vi "Camber controller April 18 2016.vi"() -> ()   [LabVIEW 2014]
uses:
  <vilib>/Utility/error.llb/DialogType.ctl
  <vilib>/Instr/_visa.llb/VISA Configure Serial Port (Instr).vi
  <vilib>/Utility/file.llb/Write To Spreadsheet File (string).vi
  <vilib>/Utility/file.llb/Write To Spreadsheet File (DBL).vi
  <vilib>/Utility/file.llb/Read From Spreadsheet File (string).vi
  <vilib>/DAQmx/read.llb/DAQmx Read (Analog 1D DBL NChan 1Samp).vi
  <vilib>/DAQmx/write.llb/DAQmx Write (Analog 1D DBL NChan 1Samp).vi
  <vilib>/DAQmx/write.llb/DAQmx Write (Digital Bool 1Line 1Point).vi
  Environmental Chamber LabVIEW and Instruments/Drivers and Software/keithley_6430/Keithley 6430/Public/Data/Read (Single Point).vi
  Environmental Chamber LabVIEW and Instruments/Drivers and Software/LabVIEW 8.2 Drivers/keithley_24xx/Keithley 24XX/Public/Data/Read (Single Point).vi
  Environmental Chamber LabVIEW and Instruments/Drivers and Software/keithley_24xx/Keithley 24XX/Keithley 24XX.lvlib
  Environmental Chamber LabVIEW and Instruments/Drivers and Software/keithley_6430/Keithley 6430/Keithley 6430.lvlib
  LabVIEW QCM code version 4 Working/(SubVI)2 2QCM.vi
  LabVIEW QCM code version 4 Working/(SubVI)1 3QCM.vi
  LabVIEW QCM code version 4 Working/(SubVI)2 3QCM.vi
  LabVIEW QCM code version 4 Working/(SubVI)1 4QCM.vi
  LabVIEW QCM code version 4 Working/(SubVI)2 4QCM.vi
  LabVIEW QCM code version 4 Working/(SubVI)1 5QCM.vi
  LabVIEW QCM code version 4 Working/(SubVI)2 5QCM.vi
  LabVIEW QCM code version 4 Working/(SubVI)1 6QCM.vi
  LabVIEW QCM code version 4 Working/(SubVI)2 6QCM.vi
panel:
  out "Sequence\npreview":cluster{dbl[], dbl[]}[](graph)
  in  "Gate time":u16(ring)=1 items=["0.1 seconds", "1.0 seconds", "10.0 seconds"]
  out "Hz":dbl format="%.2f"
  out "Waveform Chart 2":T1(graph)
  in  "User-defined\nsequence":string[][](table) caption="Create sequence"
  out "Sequence end time":string
  in  "Run Sequence":bool
  in  "Import sequence file":bool
  in  "Save sequence":bool
  in  "Clear sequence":bool
  out "arduino qcm 6":cluster{"Mean":dbl}(graph)
  out "arduino qcm 5":cluster{"Mean":dbl}(graph)
  out "arduino qcm 4":cluster{"Mean":dbl}(graph)
  out "arduino qcm 1":cluster{"Mean":dbl}(graph)
  out "arduino qcm 3":cluster{"Mean":dbl}(graph)
  out "arduino qcm 2":cluster{"Mean":dbl}(graph)
  in  "electrical/optical tab":enum32{"Electrical", "Optical"}(tab)
  out "Keithley 6430 (Ohm)":cluster{"Measurement":dbl}(graph)
  out "Keithley 2420 (Ohm)":cluster{"Resistance":sgl}(graph)
  in  "Seconds between  spectra":dbl caption="Time Target (s)"
  in  "Save spectra file path":path=path "C:/Users/User/Desktop/Chamber Data/perovskites/2015-08-04 spectra"
  in  "spectra settings":i32[](array[numeric]) caption="Integration time (ms)\n\nOptical smoothing level\n\nNumber of scans to average\n\nDigitizer clock rate setting" min=0 max=4 step=1
  in  "Aquire spectra":bool
  out "Critical Error":bool
  out "output param":i32
  out "Spectrum":cluster{"Wavelengths":dbl[], "buffer out":sgl[]}(graph)
  in  "Analyte part. press. (%)":dbl=100.0 min=0.0 max=100.0 step=5.0
  in  "Pressure Mode":T2(radio)
  in  "Turbo pump auto on":bool=TRUE
  in  "Gas sccm":sgl min=0 max=200 step=5
  out "Actual vapor flow":dbl format="%#_3g"
  out "actual gas flow":dbl format="%#_3g"
  in  "Vapor sccm":sgl min=0 max=200 step=5
  in  "Valve":enum32{"% Open", "Torr "}(radio)
  out "Valve position (%)":dbl format="%#_2f"
  in  "Desired pressure":dbl min=0.0 max=760.0 step=5.0
  in  "valve % open":dbl=100.0 min=0.0 max=100.0 step=5.0 format="%#_2f"
  out "actual pressure":dbl format="%#_3g"
  out "Currently saving data":bool
  in  "Data saving":T3(radio)
  out "J-Kem Temp (C)":cluster{"Numeric Control":dbl}(graph)
  out "Chamber Pressure (Torr)":cluster{"f":dbl}(graph)
  in  "Start saving after":dbl caption="min"
  in  "Auto stop after":bool
  in  "hrs":dbl=1000.0 min=0.0
  out "Start Time":string
  out "Elapsed (min)":dbl caption="Elapsed Time (s)" format="%#_4g"
  in  "Delay between data points (s)":dbl caption="sec" min=0.0 max=30.0 format="%#_13g"
  in  "stop":bool
  in  "Experiment Notes":string
  in  "Clear all charts":bool
  out "Data file save path":path
  out "Array for Mean 7":dbl[](array[numeric]) format="%#_8g"
  out "Array for Median 7":dbl[](array[numeric]) format="%#_8g"
  out "Mean 7":dbl format="%#_8g"
  out "Median 7":dbl format="%#_8g"
  out "Array for Mean 6":dbl[](array[numeric]) format="%#_8g"
  out "Array for Median 6":dbl[](array[numeric]) format="%#_8g"
  out "Mean 6":dbl format="%#_8g"
  out "Median 6":dbl format="%#_8g"
  out "Array for Mean 5":dbl[](array[numeric]) format="%#_8g"
  out "Array for Median 5":dbl[](array[numeric]) format="%#_8g"
  out "Mean 5":dbl format="%#_8g"
  out "Median 5":dbl format="%#_8g"
  out "Array for Mean 4":dbl[](array[numeric]) format="%#_8g"
  out "Array for Median 4":dbl[](array[numeric]) format="%#_8g"
  out "Mean 4":dbl format="%#_8g"
  out "Median 4":dbl format="%#_8g"
  out "Array for Mean 3":dbl[](array[numeric]) format="%#_8g"
  out "Array for Median 3":dbl[](array[numeric]) format="%#_8g"
  out "Mean 3":dbl format="%#_8g"
  out "Median 3":dbl format="%#_8g"
  out "Array for Mean 2":dbl[](array[numeric]) format="%#_8g"
  out "Array for Median 2":dbl[](array[numeric]) format="%#_8g"
  out "Mean 2":dbl format="%#_8g"
  out "Median 2":dbl format="%#_8g"
  out "appended array":dbl[](array[numeric]) caption="atm\nTorr"
  in  "rapidox O2 Sensor":bool
  in  "setnag O2 Pump":bool
  in  "Baud Rate 2":i32(ring)=2 items=["2400", "4800", "9600", "19200", "38400", "57600", "115200"]
  in  "Com Port":i32(ring) items=["Com 1", "Com 2", "Com 3", "Com 4", "Com 5", "Com 6", "COM 7", "COM 8", "COM 9", "COM 10", "COM 11", "COM 12", "com 13", "COM 14"]
  in  "Com Port 2":i32(ring) items=["Com 1", "Com 2", "Com 3", "Com 4", "Com 5", "Com 6", "COM 7", "COM 8", "COM 9", "COM 10", "COM 11", "COM 12", "com 13", "COM 14"]
  out "Waveform Chart":cluster{dbl}(graph)
  out "O2 Concentration (PPM)":dbl
  out "Waveform Chart 6":cluster{dbl}(graph)
  # "Currently Unused"
  # "Gas/Vapor Sequence"
  # "Pressure Control"
  # "Actual"
  # "Set"
  # "SRS QCM"
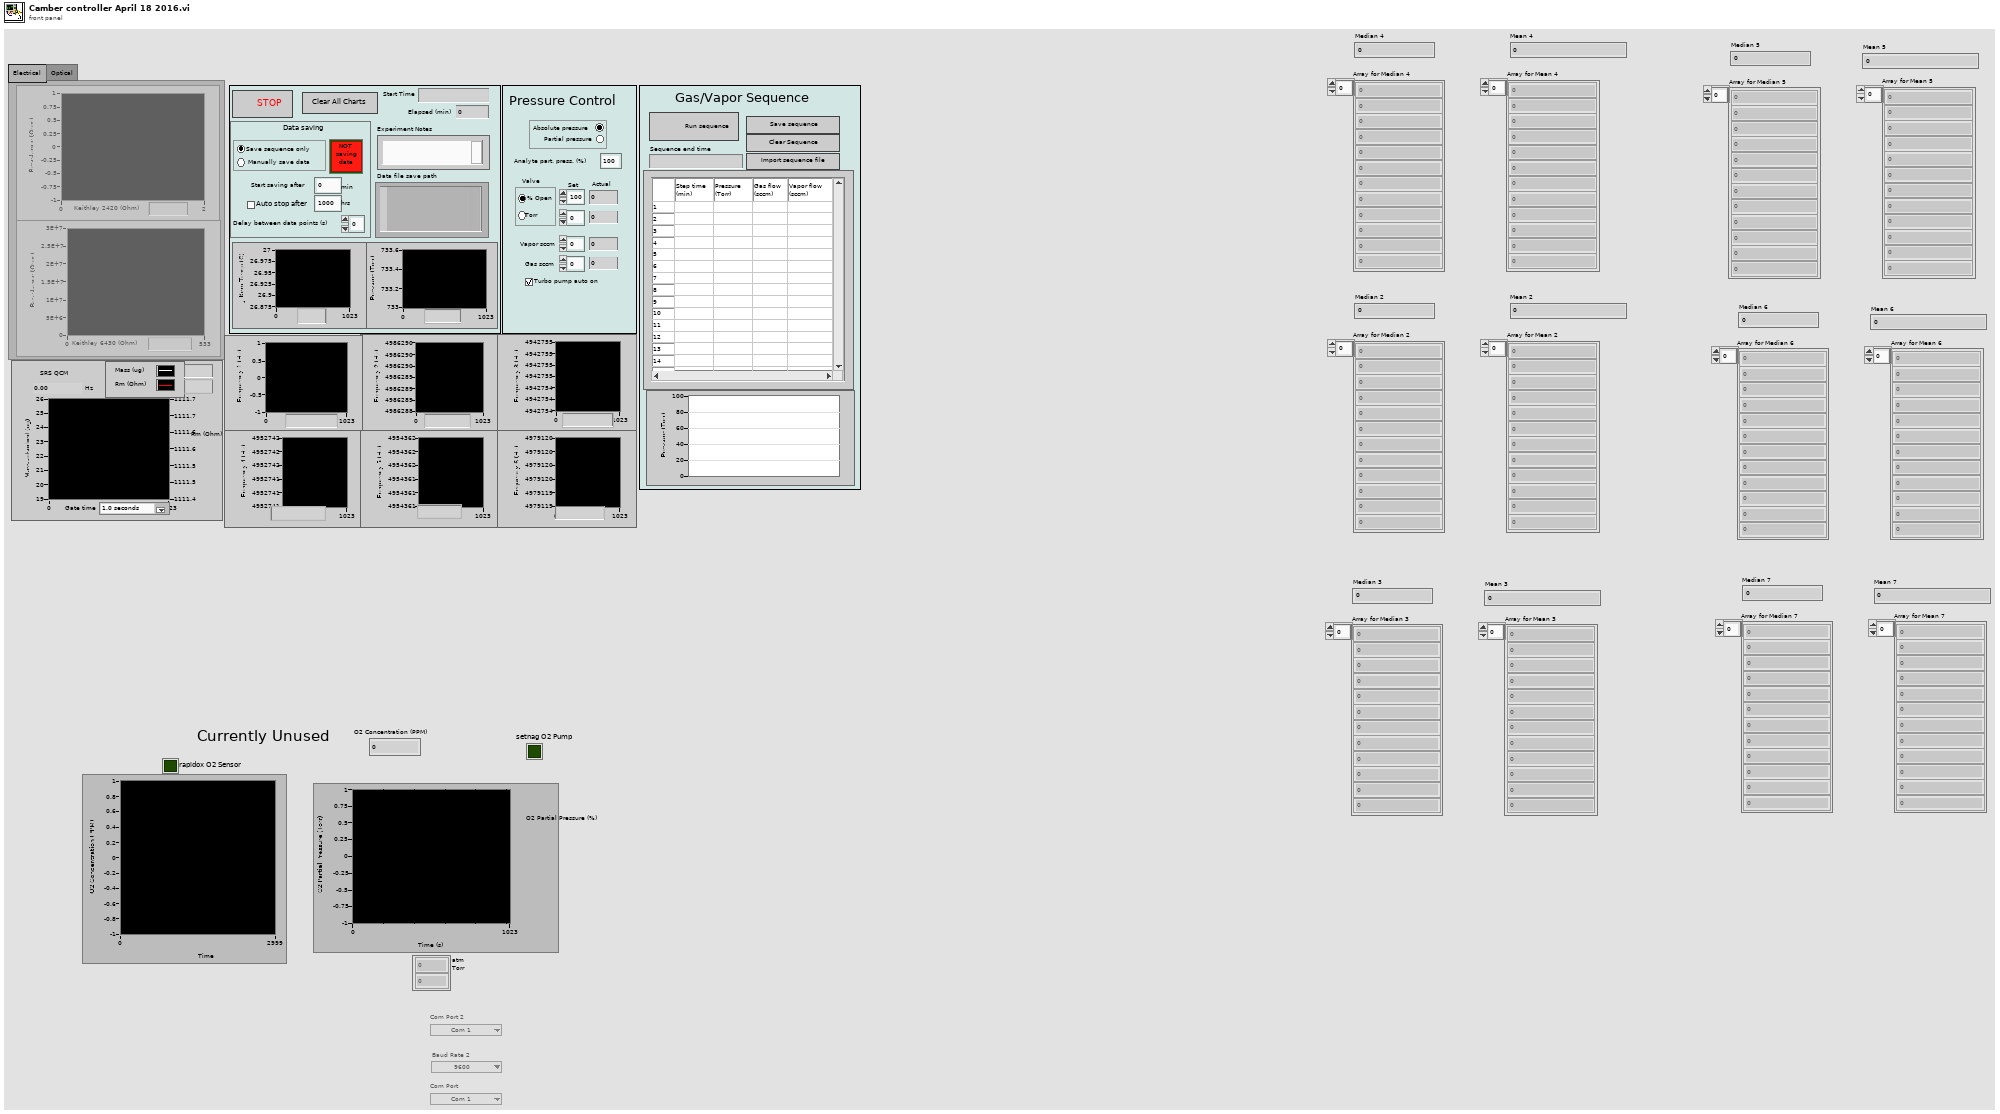
[diagram p1: front panel]
types:
  T1 = cluster{"Numeric Control":dbl, "Resistance out":dbl}
  T2 = enum32{"Absolute pressure ", " Partial pressure"}
  T3 = enum32{"Save sequence only", " Manually save data"}
  T4 = enum16{"open", "open or create", "create or replace", "create", "open (read only)"}
  T5 = enum8{"Enabled", "Disabled", "Disabled and Grayed Out"}
  T6 = enum16{"no parity", "odd parity", "even parity", "mark parity", "space parity"}
  T7 = cluster{"task out":refnum<k21>, "error out":errorcluster, "task out":refnum<k21>, "error out":errorcluster, "task out":refnum<k21>, "error out":errorcluster, "VISA resource name":refnum<visa-resource-name>, "error out":errorcluster}
  T8 = cluster{"task out":refnum<k21>, "error out":errorcluster, "task out":refnum<k21>, "error out":errorcluster, "task out":refnum<k21>, "error out":errorcluster, "VISA resource name out":refnum<visa-resource-name>, "error out":errorcluster}
  T9 = cluster{bool, "VISA resource name":refnum<visa-resource-name>, "error out":errorcluster}
  T10 = cluster{bool, "VISA resource name out":refnum<visa-resource-name>, "error out":errorcluster}
  T11 = cluster{"Boolean":bool, "VISA resource name out":refnum<visa-resource-name>, "error out":errorcluster}
  T12 = cluster{"Coefficients":ext[], "Wavelengths":dbl[]}[]
  T13 = cluster{"Integration Time (ms)":i32, "Number of Scans to Average":i32, "Optical Smoothing Level":i32, "Digitizer Clock Rate Setting":i32, "Temp  Compensation ":bool}[]
  T14 = cluster{"Integration Time (ms)":i32, "Number of Scans to Average":i32, "Optical Smoothing Level":i32, "Digitizer Clock Rate Setting":i32, "Temp  Compensation ":bool}
  T15 = cluster{"Coefficients":ext[], "Wavelengths":dbl[]}
  T16 = cluster{bool, "VISA out":refnum<visa-resource-name>, "error out":errorcluster}
  T17 = cluster{"Boolean":bool, "VISA out":refnum<visa-resource-name>, "error out":errorcluster}
  T18 = cluster{"date/time string":string, "save elapsed time":string}
  T19 = typedef "DialogType.ctl" = u16
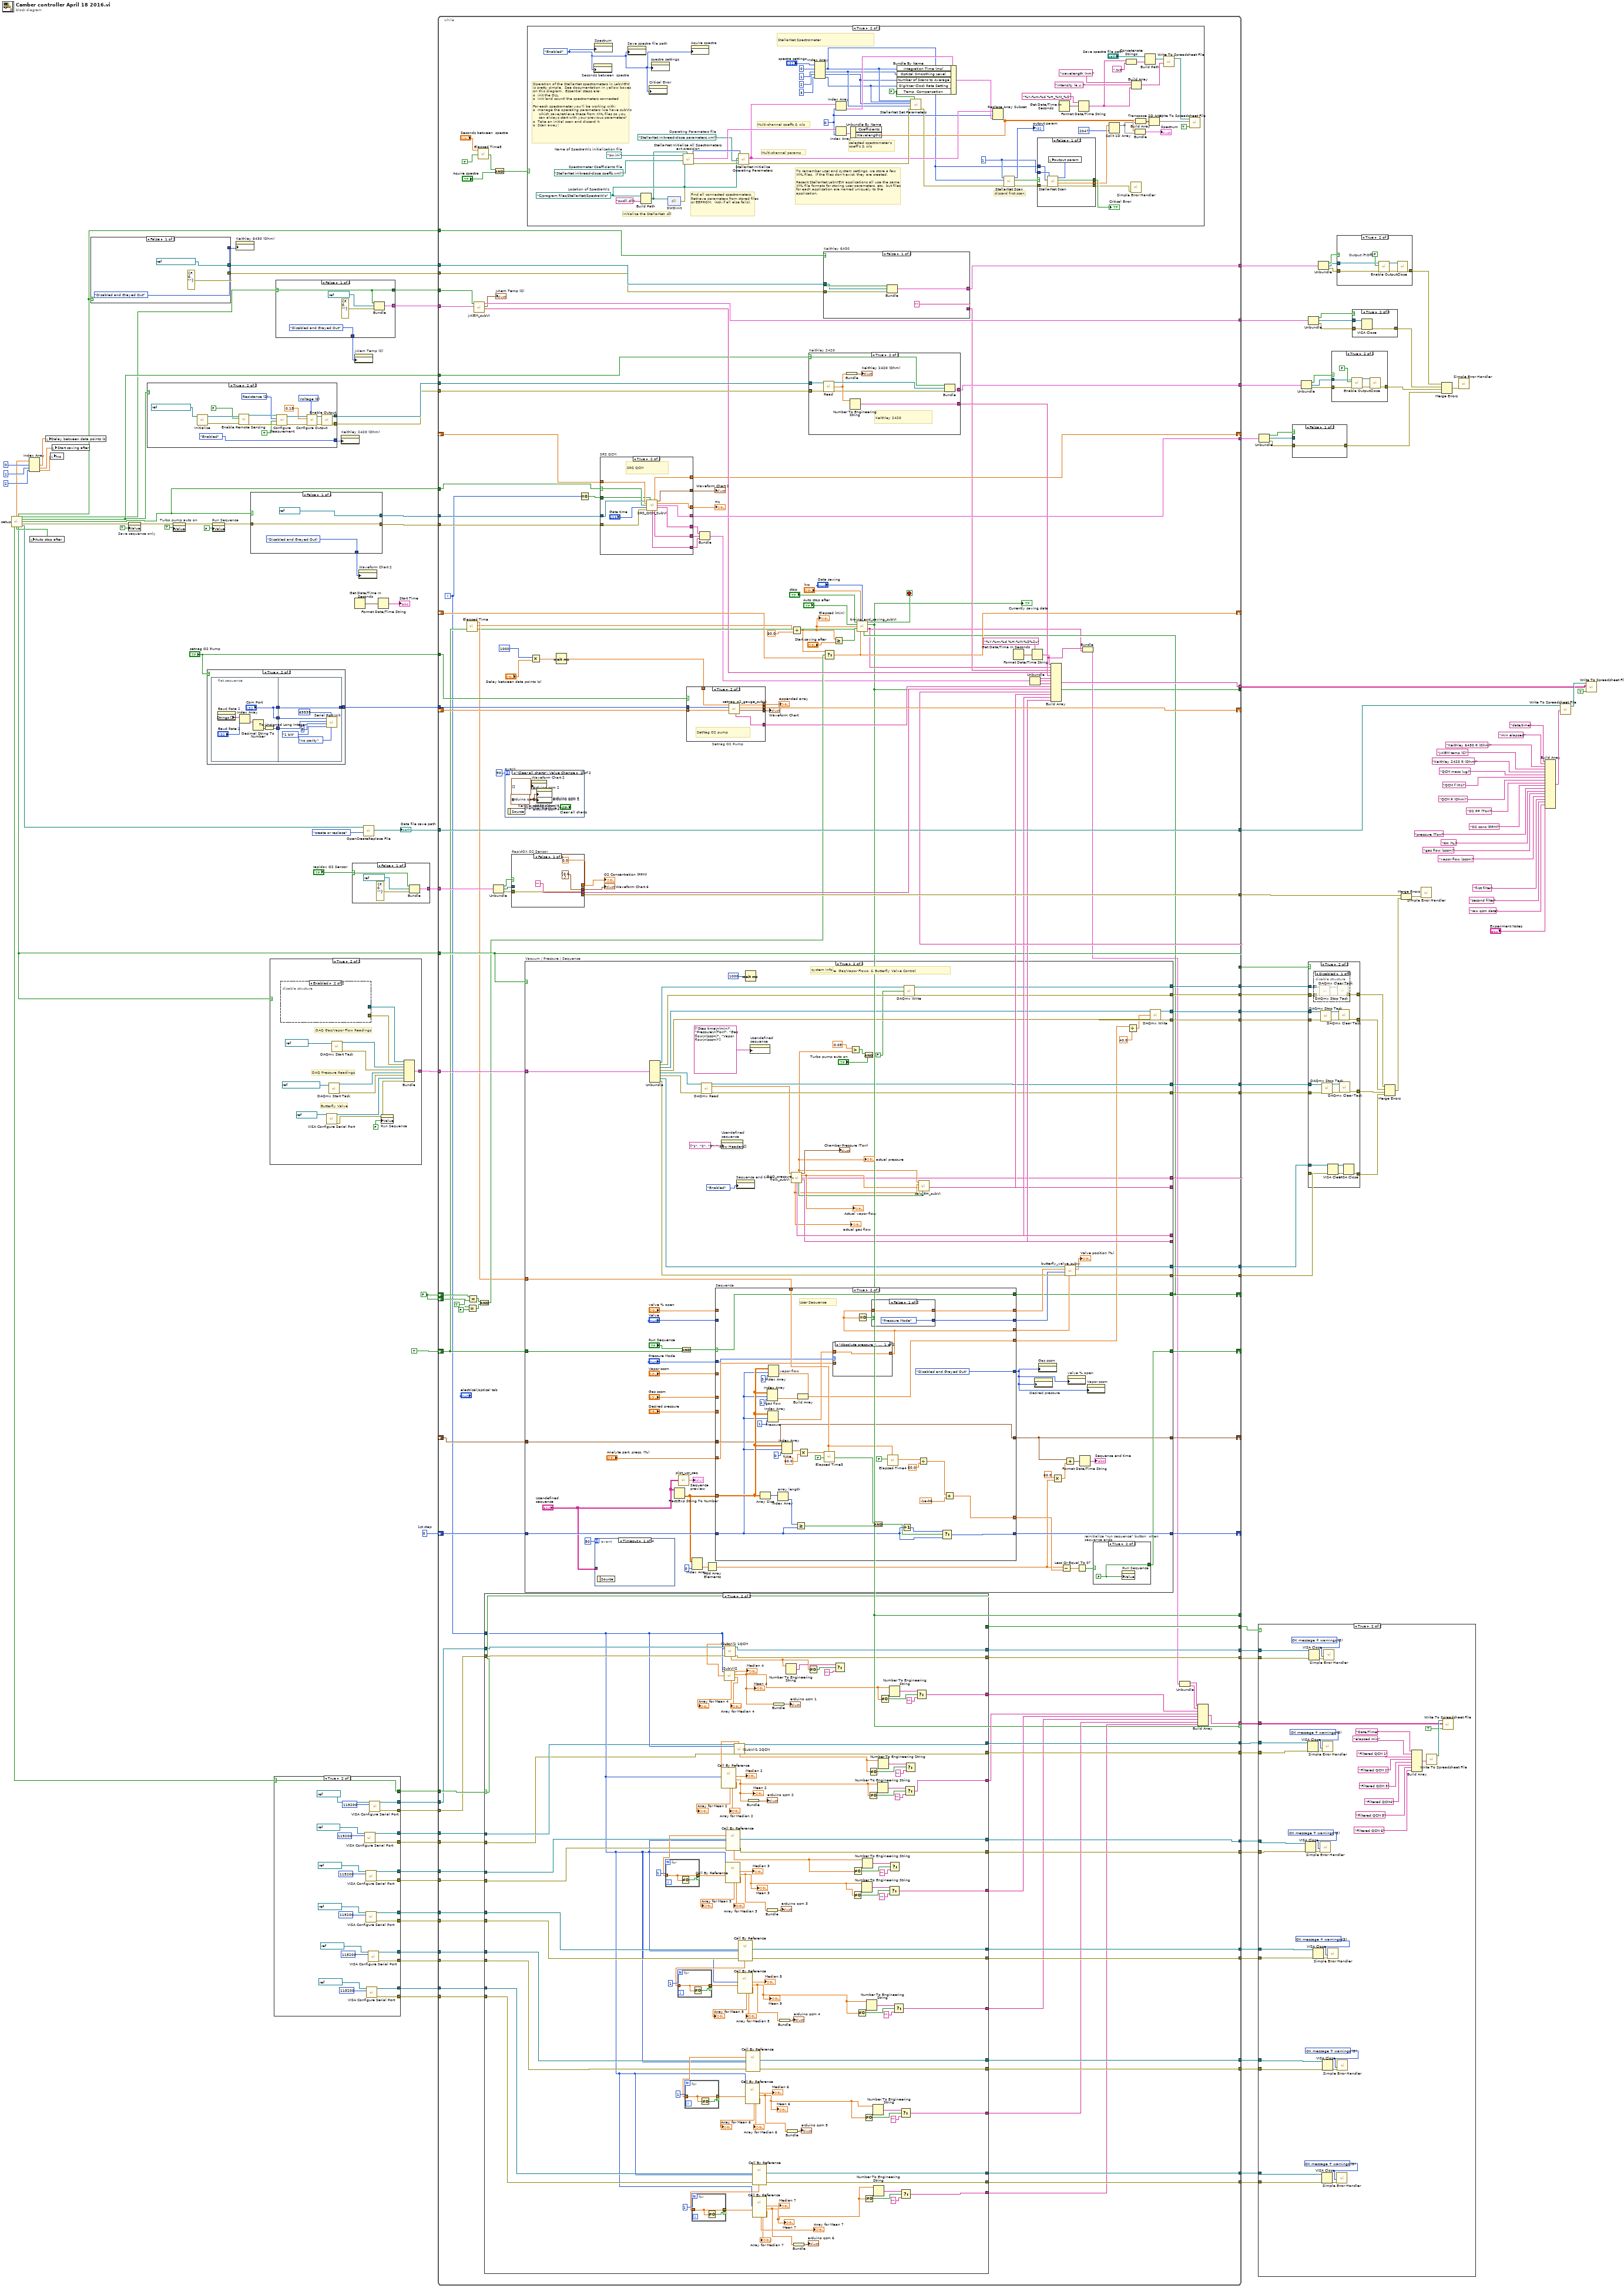
[diagram p0: block diagram]
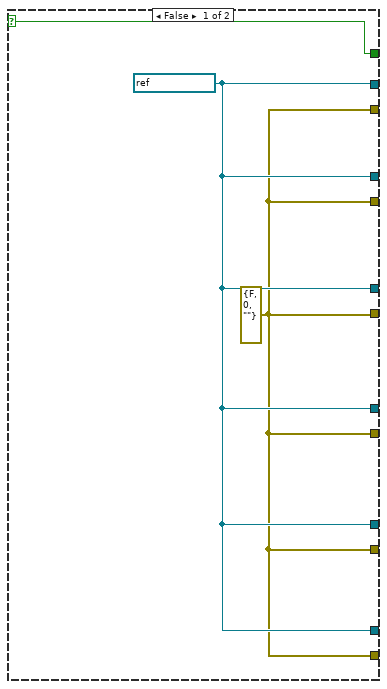
[diagram p2: hidden frame]
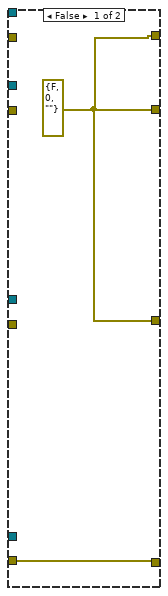
[diagram p4: hidden frame]
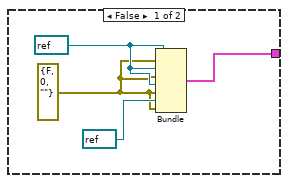
[diagram p6: hidden frame]
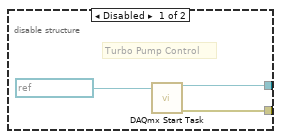
[diagram p7: hidden frame]
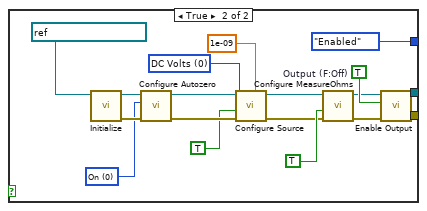
[diagram p9: hidden frame]
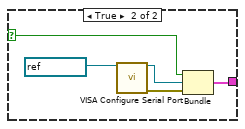
[diagram p10: hidden frame]
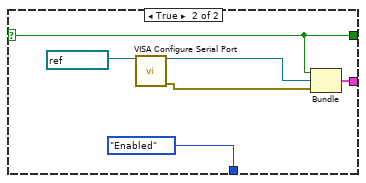
[diagram p12: hidden frame]
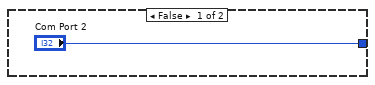
[diagram p13: hidden frame]
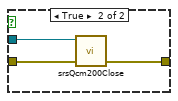
[diagram p14: hidden frame]
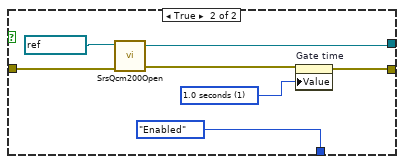
[diagram p15: hidden frame]
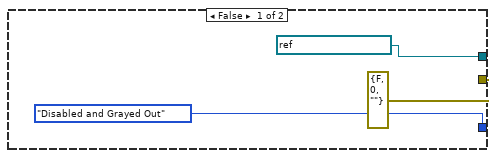
[diagram p17: hidden frame]
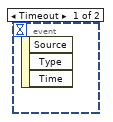
[diagram p18: hidden frame]
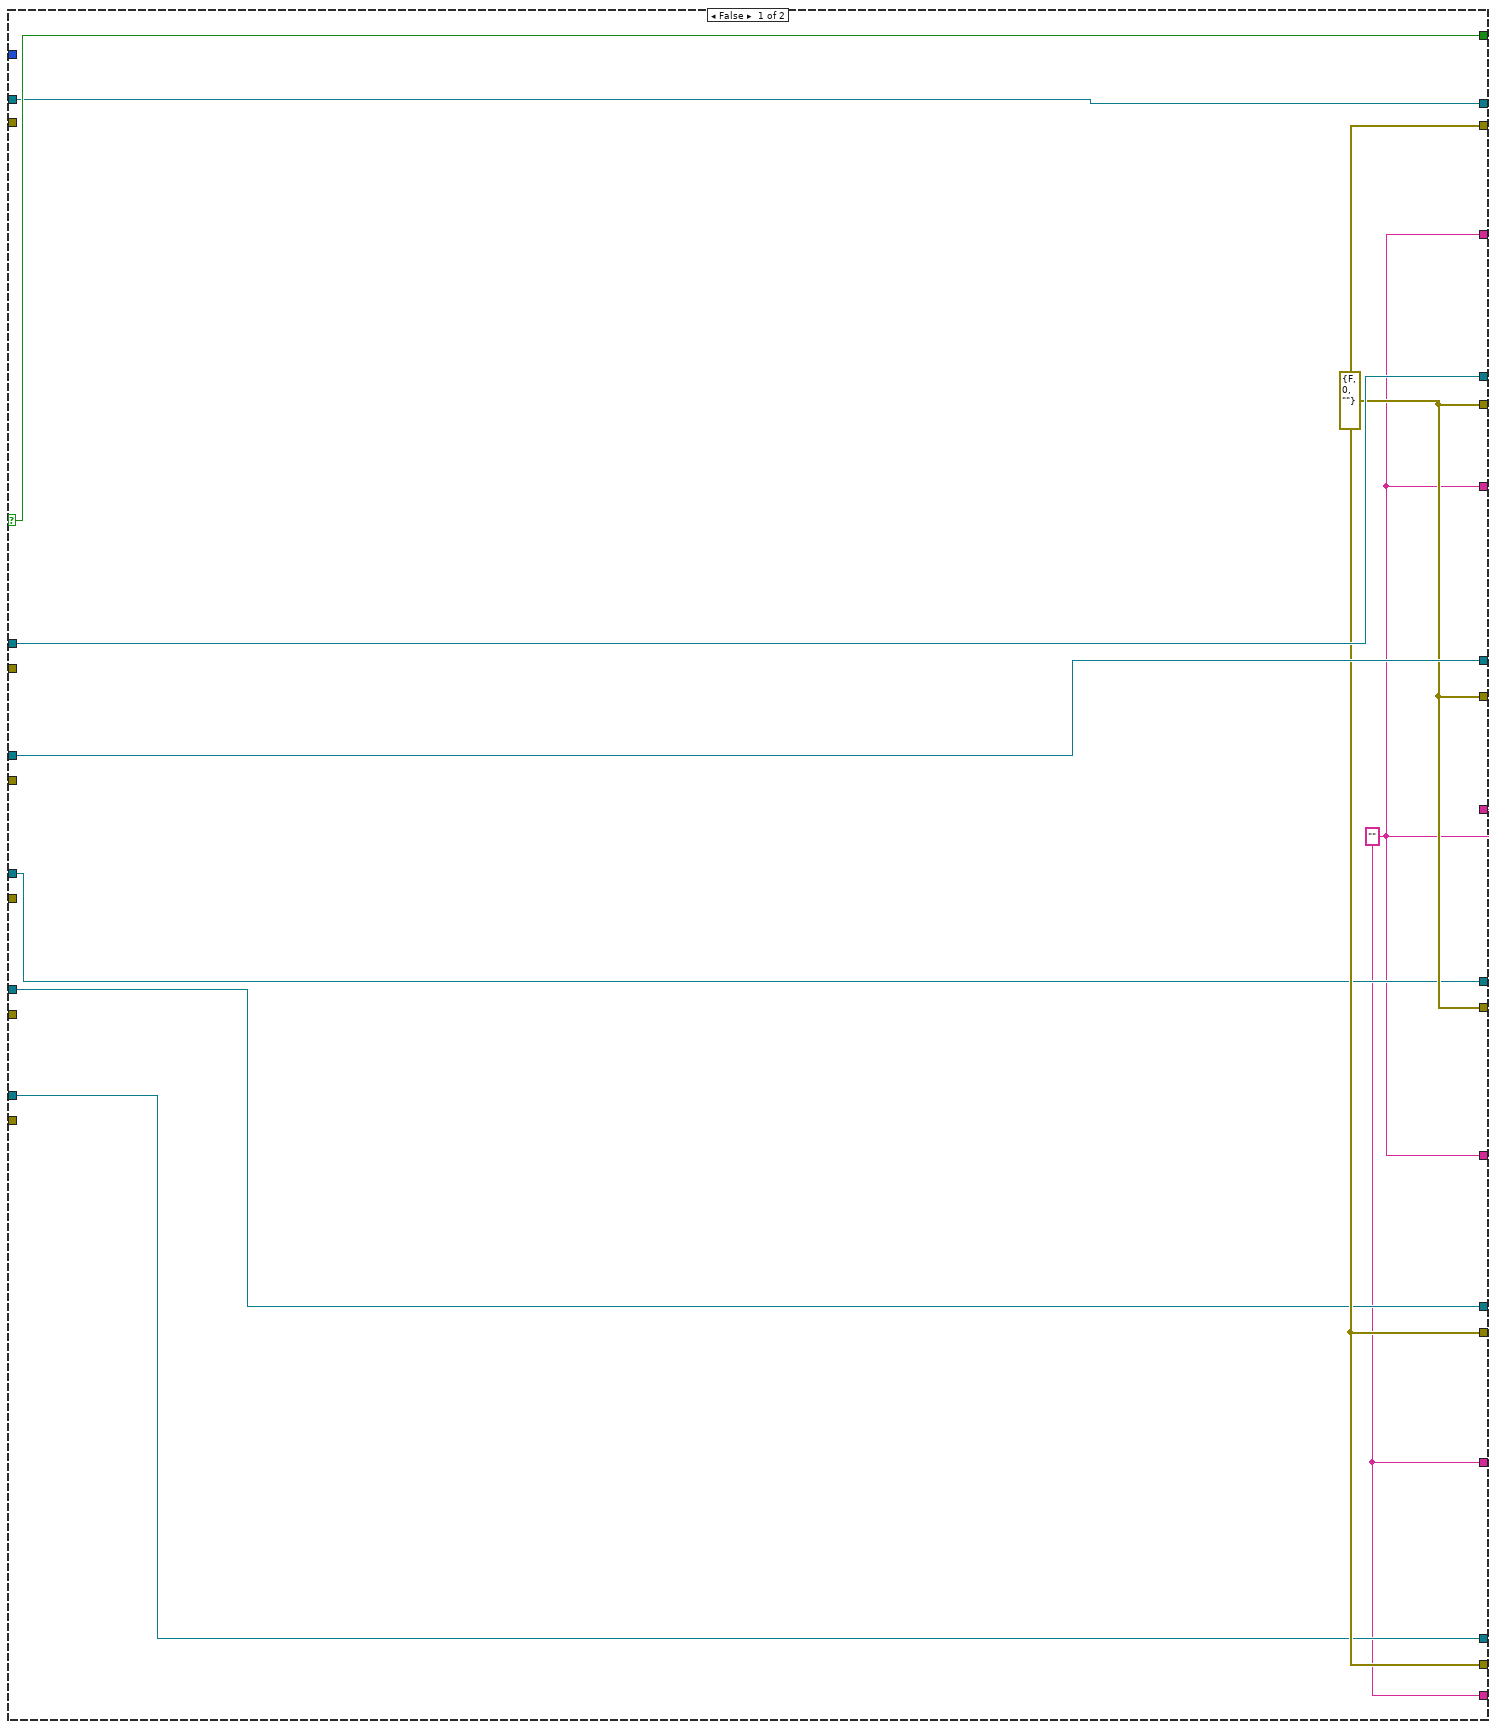
[diagram p19: hidden frame]
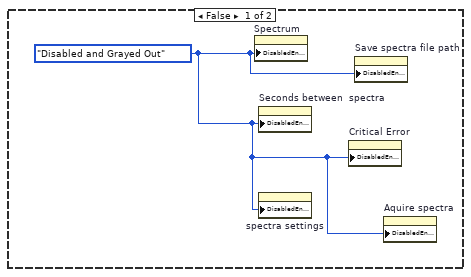
[diagram p20: hidden frame]
diagram:
  w34 = FALSE ("new element/subarray")
  w66 = 0  # 1st step
  n1 = call "setup.vi"() -> ("delay, begin, stop settings 2"=w49:dbl[], "Keithley 6431"=w41:bool, "J-KEM2"=w39:bool, "Keithley 2421"=w40:bool, "SRS QCM 2"=w44:bool, "error IO"=w14:errorcluster, "Arduino2"=w27:bool, "Auto Stop 2"=w45:bool, "Pressure control 2"=w42:bool, "Save file path 2"=w43:path)  [unwired: 6 in]
  n2 = Index Array(array=w49, index #1=0 ("index"), index #2=1 ("index"), index #3=2 ("index")) -> (element #1=w48:dbl, element #2=w47:dbl, element #3=w46:dbl)
  n3 = local write "Auto stop after"(w45) -> ()
  n4 = local write "Delay between data points (s)"(w48) -> ()
  n5 = local write "hrs"(w46) -> ()
  n6 = local write "Start saving after"(w47) -> ()
  n7 = case shown="False" w41 {
    tunnel: [refnum<visa-resource-name> "GPIB0::29::INSTR" ("VISA resource name") w149] -> w89
    tunnel: [errorcluster {"status"=FALSE, "code"=0, "source"=""} ("error out") w150] -> w88
    tunnel: [T5."Disabled and Grayed Out" ("Disabled") T5."Enabled" ("Disabled")] -> w35
    frame False {
    }
    frame True {
      w138 = u16 0 items=["DC Volts", "DC Current"] ("Source Function (0: DC Volts)")
      w145 = u16 0 items=["On", "Off", "Once"] ("Autozero  (0: On)")
      w153 = TRUE  # Output (F:Off)
      n8 = call "Initialize.vi"("VISA resource name"=refnum<visa-resource-name> "GPIB0::29::INSTR") -> ("error out"=w146:errorcluster, "VISA resource name out"=w147:refnum<visa-resource-name>)  [unwired: 4 in, 5 out]
      n9 = call "Configure Autozero.vi"("error in (no error)"=w146, "Autozero  (0: On)"=w145, "VISA resource name"=w147) -> ("error out"=w141:errorcluster, "VISA resource name out"=w143:refnum<visa-resource-name>)  [unwired: 7 in]
      n10 = call "Configure Source.vi"("I-Source Level [A]"=1e-09, "error in (no error)"=w141, "Auto Range (T:Enable)"=TRUE, "Source Function (0: DC Volts)"=w138, "VISA resource name"=w143) -> ("error out"=w140:errorcluster, "VISA resource name out"=w142:refnum<visa-resource-name>)  [unwired: 5 in]
      n11 = call "Configure MeasureOhms.vi"("error in (no error)"=w140, "Auto Range (T:Enable)"=TRUE, "VISA resource name"=w142) -> ("error out"=w154:errorcluster, "VISA resource name out"=w152:refnum<visa-resource-name>)  [unwired: 3 in, 4 out]
      n12 = call "Enable Output.vi"("error in (no error)"=w154, "Enable Output (F:Off)"=w153, "VISA resource name"=w152) -> ("error out"=w150:errorcluster, "VISA resource name out"=w149:refnum<visa-resource-name>)  [unwired: 7 out]
    }
  }
  n13 = property on="Save sequence only" class="Bool (strict)"(error in=w14, "Value"=TRUE) -> (error out=w32:errorcluster)  [unwired: 1 in, 1 out]
  n14 = case shown="True" w40 {
    tunnel: [refnum<visa-resource-name> "GPIB1::24::INSTR" ("VISA resource name") w166] -> w131
    tunnel: [errorcluster {"status"=FALSE, "code"=0, "source"=""} ("error out") w161] -> w130
    tunnel: [T5."Disabled and Grayed Out" ("Disabled") T5."Enabled" ("Disabled")] -> w37
    frame False {
    }
    frame True {
      w168 = u16 0 items=["Voltage", "Current"] ("Source Mode  (0: Voltage)")
      w173 = u16 2 items=["Volts", "Current", "Resistance"] ("Function (0: Volts)")
      n15 = call "Initialize.vi"("VISA resource name"=refnum<visa-resource-name> "GPIB1::24::INSTR") -> ("error out"=w162:errorcluster, "VISA resource name out"=w165:refnum<visa-resource-name>)  [unwired: 9 in]
      n16 = call "Enable Remote Sensing.vi"("error in (no error)"=w162, "Enable Remote Sensing (T: Enable)"=FALSE ("4-wire?"), "VISA resource name"=w165) -> ("error out"=w163:errorcluster, "VISA resource name out"=w164:refnum<visa-resource-name>)  [unwired: 7 in]
      n17 = call "Configure Measurement.vi"("error in (no error)"=w163, "Enable Auto Range (T:Enable)"=TRUE, "Function (0: Volts)"=w173, "VISA resource name"=w164) -> ("error out"=w172:errorcluster, "VISA resource name out"=w171:refnum<visa-resource-name>)  [unwired: 6 in]
      n18 = call "Configure Output.vi"("Source Mode  (0: Voltage)"=w168, "error in (no error)"=w172, "Output Level (0)"=0.15 ("Applied Voltage (V)"), "VISA resource name"=w171) -> ("error out"=w170:errorcluster, "VISA resource name out"=w169:refnum<visa-resource-name>)  [unwired: 6 in]
      n19 = call "Enable Output.vi"("error in (no error)"=w170, "VISA resource name"=w169) -> ("error out"=w161:errorcluster, "VISA resource name out"=w166:refnum<visa-resource-name>)  [unwired: 8 in]
    }
  }
  n20 = property on="Turbo pump auto on" class="Bool (strict)"(error in=w32, "Value"=TRUE ("Turbo\npump")) -> (error out=w57:errorcluster)  [unwired: 1 in, 1 out]
  n21 = case shown="True" "setnag O2 Pump" {
    tunnel: ["Com Port 2" w176] -> w127
    frame False {
    }
    frame True {
      n22 = flat-sequence {
        tunnel: ["Com Port"] -> w179
        tunnel: [w181] -> w178
        tunnel: ["Com Port"] -> w177
        tunnel: w179 -> [w187]
        tunnel: w178 -> [w186]
        tunnel: w177 -> [w188]
        tunnel: [w188] -> w176
        frame #0 {
          n23 = property on="Baud Rate 2" class="Ring (strict)"() -> ("Strings []"=w183:string[])  [unwired: 2 in, 2 out]
          n24 = Index Array(array=w183, index="Baud Rate 2") -> (element=w184:string)
          n25 = Decimal String To Number(string=w184) -> (number=w182:i32)  [unwired: 2 in, 1 out]
          n26 = To Unsigned Long Integer(number=w182) -> (unsigned 32bit integer=w181:u32)
        }
        frame #1 {
          n27 = call <vilib>:"Serial Port Init.vi"("parity"=T6."no parity", "buffer size"=u16 65535, "stop bits"=enum16{"1 bit", "1.5 bits", "2 bits"}."1 bit", "data bits"=u16 8, "baud rate"=w186, "port number"=w187) -> ()  [unwired: 1 in, 1 out]
        }
      }
    }
  }
  n28 = property on="Run Sequence" class="Bool (strict)"(error in=w57, "Value"=FALSE ("Run Sequence")) -> (error out=w60:errorcluster)  [unwired: 1 in, 1 out]
  n29 = property on="Keithley 6430 (Ohm)" class="WFChart (strict)"("DisabledEnum"=w35) -> ()  [unwired: 2 in, 2 out]
  n30 = case shown="False" w44 {
    tunnel: [refnum<visa-resource-name> "COM6" ("VISA in") w199] -> w129
    tunnel: [w194 w196] -> w128
    tunnel: w60 -> [w194 w201]
    tunnel: [T5."Disabled and Grayed Out" ("Disabled") T5."Enabled" ("Disabled")] -> w38
    frame False {
    }
    frame True {
      w198 = u16 1 items=["0.1 seconds", "1.0 seconds", "10.0 seconds"] ("Gate time")
      n31 = call "SrsQcm200Open.vi"("error in"=w201, "VISA in"=refnum<visa-resource-name> "COM6") -> ("error out"=w197:errorcluster, "VISA out"=w199:refnum<visa-resource-name>)  [unwired: 3 in]
      n32 = property on="Gate time" class="Ring (strict)"(error in=w197, "Value"=w198) -> (error out=w196:errorcluster)  [unwired: 1 in, 1 out]
    }
  }
  n33 = case shown="True" w42 {
    tunnel: [w203 w210] -> w71
    frame False {
      w205 = refnum<k21> refnum ("task out")
      w204 = errorcluster {"status"=FALSE, "code"=0, "source"=""} ("error out")
      n34 = Bundle("task out"=w205, "error out"=w204, "task out"=w205, "error out"=w204, "task out"=w205, "error out"=w204, "VISA resource name"=refnum<visa-resource-name> refnum, "error out"=w204) -> (w203:T7)  [unwired: 1 in]
    }
    frame True {
      # "DAQ Gas/Vapor Flow Readings"
      # "DAQ Pressure Readings"
      # "Butterfly Valve"
      n35 = disable-structure shown="Enabled" {
        disable-tunnel: [w222 _] -> w217
        disable-tunnel: [w221 _] -> w216
        frame Disabled {
          # "Turbo Pump Control"
          n36 = call <vilib>:"DAQmx Start Task.vi"("task/channels in"=refnum<k21> "TurboON") -> ("task out"=w222:refnum<k21>, "error out"=w221:errorcluster)  [unwired: 13 in]
        }
        frame Enabled {
        }
      }
      n37 = call-poly "VISA Configure Serial Port"("VISA resource name"=refnum<visa-resource-name> "COM5") -> ("VISA resource name out"=w211:refnum<visa-resource-name>, "error out"=w207:errorcluster)  [unwired: 13 in]
      n38 = call <vilib>:"DAQmx Start Task.vi"("task/channels in"=refnum<k21> "AllDaqReadings") -> ("task out"=w213:refnum<k21>, "error out"=w212:errorcluster)  [unwired: 13 in]
      n39 = call <vilib>:"DAQmx Start Task.vi"("task/channels in"=refnum<k21> "Setflow") -> ("task out"=w215:refnum<k21>, "error out"=w214:errorcluster)  [unwired: 13 in]
      n40 = property on="Run Sequence" class="Bool (strict)"(error in=w207, "Value"=FALSE ("Run Sequence")) -> (error out=w209:errorcluster)  [unwired: 1 in, 1 out]
      n41 = Bundle("task out"=w217, "error out"=w216, "task out"=w215, "error out"=w214, "task out"=w213, "error out"=w212, "VISA resource name out"=w211, "error out"=w209) -> (w210:T8)  [unwired: 1 in]
    }
  }
  n42 = case shown="True" w27 {
    selector: w27 -> [w226 w251]
    tunnel: [w226 w251] -> w29
    tunnel: [w225 w248] -> w26
    tunnel: [w224 w247] -> w25
    tunnel: [w225 w245] -> w22
    tunnel: [w224 w244] -> w21
    tunnel: [w225 w242] -> w18
    tunnel: [w224 w241] -> w17
    tunnel: [w225 w232] -> w13
    tunnel: [w224 w231] -> w12
    tunnel: [w225 w230] -> w11
    tunnel: [w224 w229] -> w10
    tunnel: [w225 w228] -> w9
    tunnel: [w224 w227] -> w8
    frame False {
      w224 = errorcluster {"status"=FALSE, "code"=0, "source"=""} ("error out")
      w225 = refnum<visa-resource-name> refnum ("VISA resource name out")
    }
    frame True {
      n43 = call-poly "VISA Configure Serial Port"("VISA resource name"=refnum<visa-resource-name> "COM37" ("Arduino 2"), "baud rate (9600)"=u32 115200) -> ("VISA resource name out"=w245:refnum<visa-resource-name>, "error out"=w244:errorcluster)  [unwired: 12 in]
      n44 = call-poly "VISA Configure Serial Port"("VISA resource name"=refnum<visa-resource-name> "COM38" ("Arduino 3"), "baud rate (9600)"=u32 115200) -> ("VISA resource name out"=w242:refnum<visa-resource-name>, "error out"=w241:errorcluster)  [unwired: 12 in]
      n45 = call-poly "VISA Configure Serial Port"("VISA resource name"=refnum<visa-resource-name> "COM40" ("Arduino 3"), "baud rate (9600)"=u32 115200) -> ("VISA resource name out"=w232:refnum<visa-resource-name>, "error out"=w231:errorcluster)  [unwired: 12 in]
      n46 = call-poly "VISA Configure Serial Port"("VISA resource name"=refnum<visa-resource-name> "COM41" ("Arduino 3"), "baud rate (9600)"=u32 115200) -> ("VISA resource name out"=w228:refnum<visa-resource-name>, "error out"=w227:errorcluster)  [unwired: 12 in]
      n47 = call-poly "VISA Configure Serial Port"("VISA resource name"=refnum<visa-resource-name> "COM39" ("Arduino 3"), "baud rate (9600)"=u32 115200) -> ("VISA resource name out"=w230:refnum<visa-resource-name>, "error out"=w229:errorcluster)  [unwired: 12 in]
      n48 = call-poly "VISA Configure Serial Port"("VISA resource name"=refnum<visa-resource-name> "COM36" ("Arduino 1"), "baud rate (9600)"=u32 115200) -> ("VISA resource name out"=w248:refnum<visa-resource-name>, "error out"=w247:errorcluster)  [unwired: 12 in]
    }
  }
  n49 = case shown="False" w39 {
    selector: w39 -> [w253 w259]
    tunnel: [w254 w260] -> w116
    tunnel: [w253 w259] -> w110
    tunnel: [T5."Disabled and Grayed Out" ("Disabled") T5."Enabled" ("Disabled")] -> w36
    frame False {
      n50 = Bundle(w253, "VISA resource name"=refnum<visa-resource-name> "COM3", "error out"=errorcluster {"status"=FALSE, "code"=0, "source"=""}) -> (w254:T9)  [unwired: 1 in]
    }
    frame True {
      n51 = call-poly "VISA Configure Serial Port"("VISA resource name"=refnum<visa-resource-name> "COM3") -> ("VISA resource name out"=w261:refnum<visa-resource-name>, "error out"=w258:errorcluster)  [unwired: 13 in]
      n52 = Bundle(w259, "VISA resource name out"=w261, "error out"=w258) -> (w260:T10)  [unwired: 1 in]
    }
  }
  n53 = property on="Keithley 2420 (Ohm)" class="WFChart (strict)"("DisabledEnum"=w37) -> ()  [unwired: 2 in, 2 out]
  n54 = case shown="False" "rapidox O2 Sensor" {
    selector: "rapidox O2 Sensor" -> [w263 w268]
    tunnel: [w264 w269] -> w98
    frame False {
      n55 = Bundle(w263, "VISA resource name"=refnum<visa-resource-name> "COM7", "error out"=errorcluster {"status"=FALSE, "code"=0, "source"=""}) -> (w264:T9)  [unwired: 1 in]
    }
    frame True {
      n56 = call-poly "VISA Configure Serial Port"("VISA resource name"=refnum<visa-resource-name> "COM7") -> ("VISA resource name out"=w270:refnum<visa-resource-name>, "error out"=w267:errorcluster)  [unwired: 13 in]
      n57 = Bundle(w268, "VISA resource name out"=w270, "error out"=w267) -> (w269:T10)  [unwired: 1 in]
    }
  }
  n58 = Get Date/Time In Seconds() -> (seconds since 1Jan1904=w133:timestamp)
  n59 = property on="J-Kem Temp (C)" class="WFChart (strict)"("DisabledEnum"=w36) -> ()  [unwired: 2 in, 2 out]
  n60 = property on="Waveform Chart 2" class="WFChart (strict)"("DisabledEnum"=w38) -> ()  [unwired: 2 in, 2 out]
  n61 = call "OpenCreateReplace File.vi"("function (open:0)"=T4."create or replace", "file path"=w43) -> ("new file path"=w62:path)  [unwired: 6 in, 3 out]
  "Data file save path" <- w62
  n62 = Format Date/Time String(seconds (now)=w133) -> (date/time string=→"Start Time":string)  [unwired: 2 in]
  n63 = while {
    shift-right: [w410] -> _
    shift-left: _ -> [w409]
    tunnel: [w361] -> w30 mode=indexing if=w272
    tunnel: w40 -> [w384]
    tunnel: w131 -> [w408]
    tunnel: w130 -> [w407]
    tunnel: w129 -> [w406]
    tunnel: w128 -> [w405]
    tunnel: w44 -> [w404]
    tunnel: "setnag O2 Pump" -> [w398]
    tunnel: w127 -> [w403]
    tunnel: [w400] -> w124
    tunnel: [w399] -> w120
    tunnel: w116 -> [w397]
    tunnel: [w396] -> w115
    tunnel: w110 -> [w394]
    tunnel: w98 -> [w392]
    tunnel: [w387] -> w53
    tunnel: [w383] -> w96
    tunnel: w62 -> [w383]
    shift-right: [w349] -> _
    shift-left: _ -> [w350]
    tunnel: w89 -> [w382]
    tunnel: w88 -> [w381]
    tunnel: [w380] -> w87
    tunnel: w41 -> [w379]
    tunnel: w42 -> [w365]
    tunnel: [w377] -> w83
    tunnel: [w376] -> w80
    tunnel: [w375] -> w82
    tunnel: [w374] -> w81
    tunnel: [w365] -> w79
    tunnel: [w373] -> w75
    tunnel: w71 -> [w369]
    tunnel: [w368] -> w69
    tunnel: [w367] -> w68
    tunnel: [w366] -> w67
    shift-right: [w364] -> _
    shift-left: w66 -> [w363]
    shift-right: [w343] -> _
    shift-left: TRUE -> [w329]
    tunnel: [w272] -> _
    shift-right: [w322] -> _
    shift-left: w34 -> [w338]
    shift-left: w34 -> [w337]
    shift-right: [w332] -> _
    shift-left: _ -> [w334]
    shift-right: [w331] -> _
    shift-left: _ -> [w330]
    tunnel: [w272] -> _
    tunnel: w29 -> [w320]
    tunnel: [w319] -> w28
    tunnel: w26 -> [w318]
    tunnel: w25 -> [w317]
    tunnel: [w316] -> w24
    tunnel: [w315] -> w23
    tunnel: w22 -> [w313]
    tunnel: w21 -> [w312]
    tunnel: [w311] -> w20
    tunnel: [w310] -> w19
    tunnel: w18 -> [w309]
    tunnel: w17 -> [w308]
    tunnel: [w307] -> w16
    tunnel: [w306] -> w15
    tunnel: w13 -> [w304]
    tunnel: w12 -> [w303]
    tunnel: w11 -> [w302]
    tunnel: w10 -> [w301]
    tunnel: w9 -> [w300]
    tunnel: w8 -> [w299]
    tunnel: [w298] -> w7
    tunnel: [w297] -> w6
    tunnel: [w296] -> w5
    tunnel: [w295] -> w4
    tunnel: [w294] -> w3
    tunnel: [w293] -> w2
    tunnel: [w273] -> w1 mode=indexing if=w272
    i -> [w314]
    stop <- w348 stop-if-true
    n64 = call "Elapsed Time"() -> ("Present (s)"=w362:dbl, "Elapsed Time (s)"=w335:dbl)  [unwired: 12 in, 6 out]
    n65 = Equal?(x=w337, y=FALSE ("x")) -> (x = y?=w342:bool)
    n66 = Equal?(x=w338, y=TRUE ("x")) -> (x = y?=w340:bool)
    n67 = call "J-KEM_subVI.vi"("Address in"=w397, "J-KEM on?"=w394) -> ("String data out"=w395:string, "plot data out"=→"J-Kem Temp (C)":cluster{"Numeric Control":dbl}, "Address out"=w396:T11)  [unwired: 7 in]
    n68 = call "Elapsed Time5"("Time Target (s)"="Seconds between  spectra", "Auto Reset"=TRUE) -> ("Time has Elapsed"=w354:bool)  [unwired: 10 in, 7 out]
    n69 = And(x=w340, y=w342) -> (x .and. y?=w336:bool)
    n70 = case shown="True" w320 {
      selector: w320 -> [w422 w472]
      tunnel: [w422 w472] -> w319
      tunnel: w318 -> [w421 w511]
      tunnel: w317 -> [_ w512]
      tunnel: [w418 w510] -> w316
      tunnel: [w421 w509] -> w315
      tunnel: w314 -> [_ w429]
      tunnel: w313 -> [w420 w428]
      tunnel: w312 -> [_ w425]
      tunnel: [w420 w427] -> w311
      tunnel: [w418 w426] -> w310
      tunnel: w309 -> [w419 w520]
      tunnel: w308 -> [_ w519]
      tunnel: [w419 w517] -> w307
      tunnel: [w418 w516] -> w306
      tunnel: w304 -> [w417 w484]
      tunnel: w303 -> [_ w483]
      tunnel: w302 -> [w416 w482]
      tunnel: w301 -> [_ w481]
      tunnel: w300 -> [w415 w479]
      tunnel: w299 -> [_ w480]
      tunnel: [w418 w478] -> w298
      tunnel: [w417 w477] -> w297
      tunnel: [w416 w476] -> w296
      tunnel: [w418 w475] -> w295
      tunnel: [w415 w474] -> w294
      tunnel: [w418 w473] -> w293
      tunnel: [w414 w463] -> w279
      tunnel: [w414 w455] -> w278
      tunnel: [w414 w446] -> w277
      tunnel: [w414 w435] -> w274
      tunnel: [w414 w434] -> w275
      tunnel: [w414 w433] -> w276
      frame False {
        w414 = "" ("f")
        w418 = errorcluster {"status"=FALSE, "code"=0, "source"=""} ("error out")
      }
      frame True {
        n71 = call "(SubVI)1 1QCM.vi"("VISA Refnum in"=w511, "main loop iteration number"=w429, "error in (no error)"=w512) -> ("Freq out"=w430:dbl, "unfiltered freq out"=w471:dbl, "VISA Refnum out"=w509:refnum<visa-resource-name>, "error out"=w510:errorcluster)  [unwired: 11 in, 2 out]
        n72 = call "(SubVI)2.vi"("Freq in"=w430, "loop iteration number"=w429) -> ("Array 2"=→"Array for Median 4":dbl[], "Mean"=w464:dbl, "Median"=→"Median 4":dbl, "Array"=→"Array for Mean 4":dbl[])  [unwired: 6 in]
        "Mean 4" <- w464
        n73 = call-by-ref "?"("VISA Refnum in"=w520, "Numeric in"=w429, "error in (no error)"=w519) -> ("Numeric out"=w518:dbl, "t"=w448:dbl, "VISA Refnum out"=w517:refnum<visa-resource-name>, "error out"=w516:errorcluster)  [unwired: 7 in, 10 out]
        n74 = for {
          N: 1 -> [_]
          tunnel: w518 -> [w536]
          tunnel: [w536] -> w522 if=w535
          n75 = Not Equal To 0?(x=w536) -> (x != 0?=w535:bool)
        }
        n76 = call-by-ref "?"("Numeric in"=w522, "Numeric"=w429) -> ("Array 2"=→"Array for Median 3":dbl[], "Mean"=w447:dbl, "Median"=→"Median 3":dbl, "Array"=→"Array for Mean 3":dbl[])  [unwired: 8 in, 2 out]
        "Mean 3" <- w447
        n77 = call "(SubVI)1 2QCM.vi"("VISA Refnum in"=w428, "Numeric in"=w429, "error in (no error)"=w425) -> ("Numeric out"=w424:dbl, "t"=w423:dbl, "VISA Refnum out"=w427:refnum<visa-resource-name>, "error out"=w426:errorcluster)  [unwired: 5 in, 8 out]
        n78 = call-by-ref "?"("Numeric in"=w424, "Numeric"=w429) -> ("Array 2"=→"Array for Median 2":dbl[], "Mean"=w456:dbl, "Median"=→"Median 2":dbl, "Array"=→"Array for Mean 2":dbl[])  [unwired: 8 in, 2 out]
        "Mean 2" <- w456
        n79 = call-by-ref "?"("VISA Refnum in"=w484, "Numeric in"=w429, "error in (no error)"=w483) -> ("Numeric out"=w500:dbl, "VISA Refnum out"=w477:refnum<visa-resource-name>, "error out"=w478:errorcluster)  [unwired: 7 in, 11 out]
        n80 = for {
          N: 1 -> [_]
          tunnel: w500 -> [w534]
          tunnel: [w534] -> w502 if=w533
          n81 = Not Equal To 0?(x=w534) -> (x != 0?=w533:bool)
        }
        n82 = call-by-ref "?"("Numeric in"=w502, "Numeric"=w429) -> ("Array 2"=→"Array for Median 5":dbl[], "Mean"=w431:dbl, "Median"=→"Median 5":dbl, "Array"=→"Array for Mean 5":dbl[])  [unwired: 8 in, 2 out]
        "Mean 5" <- w431
        n83 = call-by-ref "?"("VISA Refnum in"=w482, "Numeric in"=w429, "error in (no error)"=w481) -> ("Numeric out"=w493:dbl, "VISA Refnum out"=w476:refnum<visa-resource-name>, "error out"=w475:errorcluster)  [unwired: 7 in, 11 out]
        n84 = for {
          N: 1 -> [_]
          tunnel: w493 -> [w532]
          tunnel: [w532] -> w495 if=w531
          n85 = Not Equal To 0?(x=w532) -> (x != 0?=w531:bool)
        }
        n86 = call-by-ref "?"("Numeric in"=w495, "Numeric"=w429) -> ("Array 2"=→"Array for Median 6":dbl[], "Mean"=w432:dbl, "Median"=→"Median 6":dbl, "Array"=→"Array for Mean 6":dbl[])  [unwired: 8 in, 2 out]
        "Mean 6" <- w432
        n87 = Bundle("Mean"=w456) -> (→"arduino qcm 2":cluster{"Mean":dbl})  [unwired: 1 in]
        n88 = call-by-ref "?"("VISA Refnum in"=w479, "Numeric in"=w429, "error in (no error)"=w480) -> ("Numeric out"=w486:dbl, "VISA Refnum out"=w474:refnum<visa-resource-name>, "error out"=w473:errorcluster)  [unwired: 7 in, 11 out]
        n89 = for {
          N: 1 -> [_]
          tunnel: w486 -> [w530]
          tunnel: [w530] -> w488 if=w529
          n90 = Not Equal To 0?(x=w530) -> (x != 0?=w529:bool)
        }
        n91 = call-by-ref "?"("Numeric in"=w488, "Numeric"=w429) -> ("Array 2"=→"Array for Median 7":dbl[], "Mean"=w436:dbl, "Median"=→"Median 7":dbl, "Array"=→"Array for Mean 7":dbl[])  [unwired: 8 in, 2 out]
        "Mean 7" <- w436
        n92 = Bundle("Mean"=w447) -> (→"arduino qcm 3":cluster{"Mean":dbl})  [unwired: 1 in]
        n93 = Bundle("Mean"=w464) -> (→"arduino qcm 1":cluster{"Mean":dbl})  [unwired: 1 in]
        n94 = Bundle("Mean"=w431) -> (→"arduino qcm 4":cluster{"Mean":dbl})  [unwired: 1 in]
        n95 = Number To Engineering String(4:w471) -> (0:w469:string)  [unwired: 3 in]
        n96 = Bundle("Mean"=w432) -> (→"arduino qcm 5":cluster{"Mean":dbl})  [unwired: 1 in]
        n97 = Bundle("Mean"=w436) -> (→"arduino qcm 6":cluster{"Mean":dbl})  [unwired: 1 in]
        n98 = Not Equal To 0?(x=w471) -> (x != 0?=w470:bool)
        n99 = Select(t=w469, s=w470, f="") -> ()  [unwired: 1 out]
        n100 = Not Equal To 0?(x=w447) -> (x != 0?=w454:bool)
        n101 = Not Equal To 0?(x=w448) -> (x != 0?=w449:bool)
        n102 = Not Equal To 0?(x=w431) -> (x != 0?=w443:bool)
        n103 = Number To Engineering String(4:w447) -> (0:w453:string)  [unwired: 3 in]
        n104 = Number To Engineering String(4:w448) -> (0:w450:string)  [unwired: 3 in]
        n105 = Not Equal To 0?(x=w432) -> (x != 0?=w442:bool)
        n106 = Not Equal To 0?(x=w436) -> (x != 0?=w437:bool)
        n107 = Number To Engineering String(4:w431) -> (0:w444:string)  [unwired: 3 in]
        n108 = Not Equal To 0?(x=w456) -> (x != 0?=w457:bool)
        n109 = Not Equal To 0?(x=w423) -> (x != 0?=w462:bool)
        n110 = Number To Engineering String(4:w432) -> (0:w441:string)  [unwired: 3 in]
        n111 = Number To Engineering String(4:w436) -> (0:w438:string)  [unwired: 3 in]
        n112 = Number To Engineering String(4:w456) -> (0:w458:string)  [unwired: 3 in]
        n113 = Number To Engineering String(4:w423) -> (0:w461:string)  [unwired: 3 in]
        n114 = Not Equal To 0?(x=w464) -> (x != 0?=w465:bool)
        n115 = Number To Engineering String(4:w464) -> (0:w466:string)  [unwired: 3 in]
        n116 = Select(t=w453, s=w454, f="") -> (s? t:f=w446:string)
        n117 = Select(t=w450, s=w449, f="") -> ()  [unwired: 1 out]
        n118 = Select(t=w444, s=w443, f="") -> (s? t:f=w433:string)
        n119 = Select(t=w441, s=w442, f="") -> (s? t:f=w434:string)
        n120 = Select(t=w438, s=w437, f="") -> (s? t:f=w435:string)
        n121 = Select(t=w458, s=w457, f="") -> (s? t:f=w455:string)
        n122 = Select(t=w461, s=w462, f="") -> ()  [unwired: 1 out]
        n123 = Select(t=w466, s=w465, f="") -> (s? t:f=w463:string)
      }
    }
    n124 = Unbundle(w392) -> (w391:bool, "VISA resource name out"=w390:refnum<visa-resource-name>, "error out"=w389:errorcluster)
    n125 = And(x=w354, y="Aquire spectra") -> (x .and. y?=w352:bool)
    n126 = event shown="[1] \"Clear all charts\": Value Change" {
      selector: _ -> [_ _]
      dyn-events: _ -> [_ _]
      timeout: 50 -> [_ _]
      event Timeout {
        n127 = event-data() -> ()  [unwired: 1 in, 3 out]
      }
      event "Clear all charts": Value Change {
        w413 = cluster{dbl}[] [] ("History Data")
        n128 = event-data() -> ()  [unwired: 1 in, 1 out]
        n129 = property on="Waveform Chart 2" class="WFChart (strict)"("History Data"=cluster{dbl, "Resistance out":dbl}[] []) -> ()  [unwired: 2 in, 2 out]
        n130 = property on="J-Kem Temp (C)" class="WFChart (strict)"("History Data"=w413) -> ()  [unwired: 2 in, 2 out]
        n131 = property on="Keithley 2420 (Ohm)" class="WFChart (strict)"("History Data"=w413) -> ()  [unwired: 2 in, 2 out]
        n132 = property on="Waveform Chart" class="WFChart (strict)"("History Data"=w413) -> ()  [unwired: 2 in, 2 out]
        n133 = property on="Waveform Chart 6" class="WFChart (strict)"("History Data"=w413) -> ()  [unwired: 2 in, 2 out]
        n134 = property on="arduino qcm 6" class="WFChart (strict)"("History Data"=w413) -> ()  [unwired: 2 in, 2 out]
        n135 = property on="arduino qcm 2" class="WFChart (strict)"("History Data"=w413) -> ()  [unwired: 2 in, 2 out]
        n136 = property on="Chamber Pressure (Torr)" class="WFChart (strict)"("History Data"=w413) -> ()  [unwired: 2 in, 2 out]
        n137 = property on="arduino qcm 5" class="WFChart (strict)"("History Data"=w413) -> ()  [unwired: 2 in, 2 out]
        n138 = property on="arduino qcm 4" class="WFChart (strict)"("History Data"=w413) -> ()  [unwired: 2 in, 2 out]
        n139 = property on="arduino qcm 3" class="WFChart (strict)"("History Data"=w413) -> ()  [unwired: 2 in, 2 out]
        n140 = property on="arduino qcm 1" class="WFChart (strict)"("History Data"=w413) -> ()  [unwired: 2 in, 2 out]
        n141 = property on="Keithley 6430 (Ohm)" class="WFChart (strict)"("History Data"=w413) -> ()  [unwired: 2 in, 2 out]
      }
    }
    n142 = case "RapidOX O2 Sensor" shown="False" w391 {
      tunnel: w390 -> [_ w784]
      tunnel: w389 -> [w777 w783]
      tunnel: ["" w782] -> w388
      tunnel: [w777 w781] -> w387
      tunnel: [0.0 w780] -> w328
      tunnel: [cluster{dbl} {0.0} w779] -> w327
      frame False {
      }
      frame True {
        # "RapidOX 2100"
        n143 = call "rapidOX_O2_sensor_subVI.vi"("error in (no error)"=w783, "VISA Refnum in"=w784) -> ("error out"=w781:errorcluster, "String"=w782:string, "Cluster"=w779:cluster{"Numeric Control":dbl}, "Numeric Control"=w780:dbl)  [unwired: 6 in]
      }
    }
    "O2 Concentration (PPM)" <- w328
    "Waveform Chart 6" <- w327
    n144 = case "Vacuum / Pressure / Sequence" shown="True" w365 {
      tunnel: [w608 w687] -> w376
      tunnel: [w609 w686] -> w374
      tunnel: [w611 w683] -> w377
      tunnel: [w610 w684] -> w375
      tunnel: [w604 w681] -> w373
      tunnel: [w605 w622] -> w372
      tunnel: [w605 w679] -> w371
      tunnel: [w605 w678] -> w370
      tunnel: w369 -> [w614 w676]
      tunnel: [w613 w667] -> w368
      tunnel: [w612 w666] -> w367
      tunnel: [w607 w665] -> w366
      tunnel: w363 -> [w606 w656]
      tunnel: [w606 w663] -> w364
      tunnel: w362 -> [_ w662]
      tunnel: w329 -> [_ w651]
      tunnel: [w603 w645] -> w343
      tunnel: [w605 w623] -> w358
      tunnel: [w603 w635] -> w322
      tunnel: [timestamp(0 s since 1904-01-01) ("seconds since 1Jan1904") w632] -> w331
      tunnel: w330 -> [_ w633]
      frame False {
        w603 = FALSE ("new element/subarray")
        w605 = ""
        n145 = property on="Sequence end time" class="Str"("DisabledEnum"=T5."Disabled and Grayed Out" ("Disabled")) -> ()  [unwired: 2 in, 2 out]
        n146 = Unbundle(w614) -> ("task out"=w613:refnum<k21>, "error out"=w612:errorcluster, "task out"=w611:refnum<k21>, "error out"=w610:errorcluster, "task out"=w608:refnum<k21>, "error out"=w609:errorcluster, "VISA resource name out"=w607:refnum<visa-resource-name>, "error out"=w604:errorcluster)
      }
      frame True {
        # "system info"
        # "DAQ Pressure, Gas/Vapor Flows, & Butterfly Valve Control"
        n147 = event shown="[0] Timeout" {
          selector: _ -> [_ _ _ _]
          dyn-events: _ -> [_ _ _ _]
          timeout: 50 -> [_ _ _ _]
          tunnel: "User-defined\nsequence" -> [_ _ w690 _]
          event Timeout {
            n148 = event-data() -> ()  [unwired: 1 in, 1 out]
          }
          event "Clear sequence": Value Change {
            n149 = event-data() -> ()  [unwired: 1 in, 1 out]
            n150 = property on="User-defined\nsequence" class="Tbl (strict)"("Value"=string[][] []) -> ()  [unwired: 2 in, 2 out]
          }
          event "Save sequence": Value Change {
            n151 = event-data() -> ()  [unwired: 1 in, 1 out]
            n152 = call-poly <vilib>:"Write To Spreadsheet File.vi"("2D data"=w690) -> ()  [unwired: 7 in, 1 out]
          }
          event "Import sequence file": Value Change {
            n153 = event-data() -> ()  [unwired: 1 in, 1 out]
            n154 = call-poly <vilib>:"Read From Spreadsheet File.vi"() -> ("all rows"=w691:string[][])  [unwired: 7 in, 4 out]
            n155 = property on="User-defined\nsequence" class="Tbl (strict)"("Value"=w691) -> ()  [unwired: 2 in, 2 out]
          }
        }
        n156 = Unbundle(w676) -> ("task out"=w669:refnum<k21>, "error out"=w668:errorcluster, "task out"=w670:refnum<k21>, "error out"=w671:errorcluster, "task out"=w672:refnum<k21>, "error out"=w673:errorcluster, "VISA resource name out"=w674:refnum<visa-resource-name>, "error out"=w675:errorcluster)
        n157 = Fract/Exp String To Number(string="User-defined\nsequence") -> (number=w650:dbl[][])  [unwired: 3 in, 1 out]
        n158 = call "plot_usr_seq.vi"("User-defined sequence"="User-defined\nsequence") -> ("Sequence Preview"=→"Sequence\npreview":cluster{dbl[], dbl[]}[])
        n159 = And(x="Run Sequence", y=w651) -> (x .and. y?=w638:bool)
        n160 = Index Array(array=w650, index (col)=0 ("disabled index (col)")) -> (element=w658:dbl[])  [unwired: 1 in]
        n161 = call-poly <vilib>:"DAQmx Read.vi"("task/channels in"=w672, "error in"=w673) -> ("task out"=w687:refnum<k21>, "data"=w685:dbl[], "error out"=w686:errorcluster)  [unwired: 11 in]
        n162 = Add Array Elements(numeric array=w658) -> (sum=w626:dbl)
        n163 = case "Sequence" shown="True" w638 {
          selector: w638 -> [w704 w730]
          tunnel: w662 -> [_ w738]
          tunnel: [w707 w739] -> w663
          tunnel: w656 -> [w707 w731]
          tunnel: "Vapor sccm" -> [w702 _]
          tunnel: "Gas sccm" -> [w701 _]
          tunnel: [w697 w715] -> w654
          tunnel: w650 -> [_ w733]
          tunnel: "Valve" -> [w706 _]
          tunnel: [w706 w726] -> w636
          tunnel: [-1e-06 w718] -> w653
          tunnel: [w704 w730] -> w635
          tunnel: [w703 w727] -> w644
          tunnel: "valve % open" -> [w703 _]
          tunnel: [w700 w723] -> w642
          tunnel: [T5."Enabled" ("Disabled") T5."Disabled and Grayed Out" ("Disabled")] -> w641
          tunnel: [w698 w721] -> w632
          tunnel: w633 -> [_ w721]
          tunnel: "Desired pressure" -> [w696 _]
          tunnel: "Pressure Mode" -> [w695 w717]
          tunnel: "Analyte part. press. (%)" -> [w694 w714]
          frame False {
            n164 = Build Array(w702, w701) -> (w700:sgl[])
            n165 = case shown="\"Absolute pressure \", Default" w695 {
              tunnel: [w708 w709] -> w697
              tunnel: w696 -> [w708 w711]
              tunnel: w694 -> [_ w710]
              frame "Absolute pressure ", Default {
              }
              frame " Partial pressure" {
                n166 = Multiply(x=w711, y=w710) -> (x*y=w713:dbl)
                n167 = Divide(x=w713, y=100.0 ("Analyte part. press. (%)")) -> (x/y=w709:dbl)
              }
            }
            n168 = Get Date/Time In Seconds() -> (seconds since 1Jan1904=w698:timestamp)
          }
          frame True {
            # "User Sequence"
            n169 = Array Size(array=w733) -> (size(s)=w750:i32[])
            n170 = Index Array "gas flow"(array=w733, index (row)=w731, index (col)=2 ("disabled index (col)")) -> (element=w724:dbl)
            n171 = Index Array "Pressure"(array=w733, index (row)=w731, index (col)=1 ("disabled index (col)")) -> (element=w716:dbl)
            n172 = Index Array "vapor flow"(array=w733, index (row)=w731, index (col)=3 ("disabled index (col)")) -> (element=w725:dbl)
            n173 = Index Array "array length"(array=w750) -> (element=w734:i32)  [unwired: 1 in]
            n174 = Index Array "time"(array=w733, index (row)=w731, index (col)=0) -> (element=w742:dbl)
            n175 = Greater Or Equal?(x=w734, y=w731) -> (x >= y?=w747:bool)
            n176 = Build Array(w725, w724) -> (w723:dbl[])
            n177 = Multiply(x=w742, y=60.0) -> (x*y=w732:dbl)
            n178 = call "Elapsed Time3"("Time Target (s)"=w732, "Auto Reset"=TRUE, "Set Start Time (s)"=w738) -> ("Time has Elapsed"=w746:bool)  [unwired: 9 in, 7 out]
            n179 = case shown="\"Absolute pressure \", Default" w717 {
              tunnel: [w751 w752] -> w715
              tunnel: w716 -> [w751 w754]
              tunnel: w714 -> [_ w753]
              frame "Absolute pressure ", Default {
              }
              frame " Partial pressure" {
                n180 = Multiply(x=w754, y=w753) -> (x*y=w755:dbl)
                n181 = Divide(x=w755, y=100.0 ("Analyte part. press. (%)")) -> (x/y=w752:dbl)
              }
            }
            n182 = Equal To 0?(x=w715) -> (x = 0?=w728:bool)
            n183 = case shown="False" w728 {
              tunnel: [enum32{"Open Mode", "Pressure Mode"}."Pressure Mode" ("Pressure Control") enum32{"Open Mode", "Pressure Mode"}."Open Mode" ("Pressure Control")] -> w726
              tunnel: [w757 100.0 ("valve % open 2")] -> w727
              tunnel: w715 -> [w757 _]
              frame False {
              }
              frame True {
              }
            }
            n184 = And(x=w746, y=w747) -> (x .and. y?=w729:bool)
            n185 = call "Elapsed Time4"("Reset"=FALSE, "Set Start Time (s)"=w738) -> ("Elapsed Time (s)"=w736:dbl)  [unwired: 10 in, 7 out]
            n186 = Increment(x=w731) -> (x+1=w740:i32)
            n187 = Divide(x=w736, y=60.0) -> (x/y=w720:dbl)
            n188 = Select(t=w740, s=w729, f=w731) -> (s? t:f=w739:i32)
            n189 = Add(x=w720, y=-1e-06) -> (x+y=w718:dbl)
          }
        }
        n190 = property on="User-defined\nsequence" class="Tbl (strict)"("Row Headers[]"=string[] ["1", "2", "3", "4", "5", "6", "7", "8", "9", "10", "11", "12", "13", "14", "15", "16", "17", "18", "19", "20", "21", "22", "23", "24", "25", "26", "27", "28", "29", "30", "31", "32", "33", "34", "35", "36", "37", "38", "39", "40"] ("Row Header Strings[]")) -> ()  [unwired: 2 in, 2 out]
        n191 = property on="Sequence end time" class="Str"("DisabledEnum"=T5."Enabled" ("Disabled")) -> ()  [unwired: 2 in, 2 out]
        n192 = Wait (ms)(milliseconds to wait=u32 1000) -> ()  [unwired: 1 out]
        n193 = property on="User-defined\nsequence" class="Tbl (strict)"("Column Headers[]"=string[] ["Step time\n(min)", "Pressure\n(Torr)", "Gas flow\n(sccm)", "Vapor flow\n(sccm)"] ("Column Header Strings[]")) -> ()  [unwired: 2 in, 2 out]
        n194 = call "DAQ_pressure_flow_subVI.vi"("vac press"=w685) -> ("low pressure"=w648:dbl, "pressure"=→"Chamber Pressure (Torr)":cluster{"f":dbl}, "vapor flow"=w624:dbl, "save pressure"=w622:string, "save pressure flow"=w678:string, "gas flow"=w634:dbl, "save gas flow"=w679:string, "both flows off?"=w649:bool)  [unwired: 6 in, 1 out]
        "actual gas flow" <- w634
        "Actual vapor flow" <- w624
        "actual pressure" <- w648
        n195 = Greater?(x=0.05, y=w648) -> (0:w659:bool)
        n196 = And(x=w659, y="Turbo pump auto on") -> ()  [unwired: 1 out]
        n197 = call-poly <vilib>:"DAQmx Write.vi"("task/channels in"=w669, "data"=FALSE, "error in"=w668) -> ("task out"=w667:refnum<k21>, "error out"=w666:errorcluster)  [unwired: 10 in, 1 out]
        n198 = call "calc_RH_subVI.vi"("Boolean"=w649, "f"=w624, "f 2"=w634, "f 3"=w648) -> ("RH"=w623:string)  [unwired: 7 in]
        n199 = property on="Desired pressure" class="DigNum (strict)"("DisabledEnum"=w641) -> ()  [unwired: 2 in, 2 out]
        n200 = property on="Gas sccm" class="DigNum (strict)"("DisabledEnum"=w641) -> ()  [unwired: 2 in, 2 out]
        n201 = Multiply(x=60.0 ("y"), y=w626) -> (x*y=w630:dbl)
        n202 = Subtract(x=w626, y=w653) -> (x-y=w637:dbl)
        n203 = call "butterfly_valve_subvi.vi"("Desired pressure"=w654, "error in (no error)"=w675, "Pressure Control"=w636, 10:w644, "VISA Refnum in"=w674) -> ("error out"=w681:errorcluster, "Valve position (%)"=→"Valve position (%)":dbl, "VISA Refnum out"=w665:refnum<visa-resource-name>)  [unwired: 4 in]
        n204 = Add(x=w632, y=w630) -> (x+y=w629:timestamp)
        n205 = property on="valve % open" class="DigNum (strict)"("DisabledEnum"=w641) -> ()  [unwired: 2 in, 2 out]
        n206 = Less Or Equal To 0?(x=w637) -> (x <= 0?=w646:bool)
        n207 = Format Date/Time String(seconds (now)=w629) -> (date/time string=→"Sequence end time":string)  [unwired: 2 in]
        n208 = property on="Vapor sccm" class="DigNum (strict)"("DisabledEnum"=w641) -> ()  [unwired: 2 in, 2 out]
        n209 = case "reinitialize \"run sequence\" button  when sequence ends" shown="True" w646 {
          tunnel: [TRUE ("Run Sequence") w693] -> w645
          frame False {
          }
          frame True {
            w693 = FALSE ("Run Sequence")
            n210 = property on="Run Sequence" class="Bool (strict)"("Value"=w693) -> ()  [unwired: 2 in, 2 out]
          }
        }
        n211 = Divide(x=w642, y=40.0 ("Waveform")) -> (x/y=w682:dbl[])
        n212 = call-poly <vilib>:"DAQmx Write.vi"("task/channels in"=w670, "data"=w682, "error in"=w671) -> ("task out"=w683:refnum<k21>, "error out"=w684:errorcluster)  [unwired: 10 in, 1 out]
      }
    }
    n213 = case shown="True" w352 {
      frame False {
        w537 = T5."Disabled and Grayed Out" ("Disabled")
        n214 = property on="Spectrum" class="XYGraph (strict)"("DisabledEnum"=w537) -> ()  [unwired: 2 in, 2 out]
        n215 = property on="Seconds between  spectra" class="DigNum (strict)"("DisabledEnum"=w537) -> ()  [unwired: 2 in, 2 out]
        n216 = property on="spectra settings" class="Arr (strict)"("DisabledEnum"=w537) -> ()  [unwired: 2 in, 2 out]
        n217 = property on="Critical Error" class="Bool (strict)"("DisabledEnum"=w537) -> ()  [unwired: 2 in, 2 out]
        n218 = property on="Save spectra file path" class="Path"("DisabledEnum"=w537) -> ()  [unwired: 2 in, 2 out]
        n219 = property on="Aquire spectra" class="Bool (strict)"("DisabledEnum"=w537) -> ()  [unwired: 2 in, 2 out]
      }
      frame True {
        w538 = T5."Enabled" ("Disabled")
        w562 = 0 ("Spectral Channel")
        w564 = 1 ("Spectral Channel")
        w568 = FALSE ("Temp  Compensation")
        w572 = path "C:/program files/StellarNet/SpectraWiz"  # Location of SpectraWiz
        w582 = path "sw.ini"  # Name of SpectraWiz initialization file
        w574 = path "StellarNet init-read-close parameters.xml"  # Operating Parameters file
        w583 = path "StellarNet init-read-close coeffs.xml"  # Spectrometer Coefficients file
        # "StellarNet Spectrometer"
        # "Operation of the StellarNet spectrometers in LabVIEW\nis pretty simple.  See documentation in yellow boxes\non this diagram.  Essential steps are:\no  init the DLL\no  init (and count) the spectrometers connected\n\nFor each spectrometer you'll be working with:\no  manage the operating parameters (we have subVIs\n     which save/retrieve these from XML files so you\n     can always start with your previous parameters)\no  Take an initial scan and discard it\no  Scan away!"
        # "initialize the StellarNet .dll"
        # "To remember user and system settings, we store a few \nXML files.  If the files don't exist, they are created.\n\nRecent StellarNet LabVIEW applications all use the same\nXML file formats for storing user parameters, etc., but files\nfor each application are named uniquely to the \napplication."
        # "Find all connected spectrometers.  Retrieve parameters from stored files or EEPROM.  (Ask if all else fails)."
        # "selected spectrometer's\ncoeff's & wls"
        # "Multi-channel coeffs & wls"
        # "Multi-channel params"
        # "discard first scan"
        n220 = property on="Seconds between  spectra" class="DigNum (strict)"("DisabledEnum"=w538) -> ()  [unwired: 2 in, 2 out]
        n221 = property on="Spectrum" class="XYGraph (strict)"("DisabledEnum"=w538) -> ()  [unwired: 2 in, 2 out]
        n222 = property on="Save spectra file path" class="Path"("DisabledEnum"=w538) -> ()  [unwired: 2 in, 2 out]
        n223 = Build Path(base path=w572, name or relative path="swdll.dll") -> (appended path=w570:path)
        n224 = property on="Critical Error" class="Bool (strict)"("DisabledEnum"=w538) -> ()  [unwired: 2 in, 2 out]
        n225 = property on="spectra settings" class="Arr (strict)"("DisabledEnum"=w538) -> ()  [unwired: 2 in, 2 out]
        n226 = dll-call lib="C:/Program Files/StellarNet/SpectraWiz/swdll.dll" fn="SWDinit" label="init"(path in=w570) -> (error out=w571:errorcluster)  [unwired: 3 in, 1 out]
        n227 = call "StellarNet Initialize All Spectrometers, ext precision.vi"("Path of swdll.dll"=w570, "error in"=w571, "Spectrometer Coefficients file"=w583, "Location of SpectraWiz"=w572, "Name of SpectraWiz initialization file"=w582) -> ("error out"=w581:errorcluster, "Multi Channel Coeffs & WLs"=w579:T12, "Number of Channels"=w580:i32)  [unwired: 2 in, 2 out]
        n228 = property on="Aquire spectra" class="Bool (strict)"("DisabledEnum"=w538) -> ()  [unwired: 2 in, 2 out]
        n229 = call "StellarNet Initialize Operating Parameters.vi"("error in"=w581, "Spectrometer Coefficients file"=w574, "Location of SpectraWiz"=w572, "Number of Channels"=w580) -> ("error out"=w577:errorcluster, "Operating Parameters"=w575:T13)  [unwired: 6 in]
        n230 = Index Array(array="spectra settings", index #1=0 ("index"), index #2=1 ("index"), index #3=2 ("index"), index #4=3 ("index")) -> (element #1=w542:i32, element #2=w541:i32, element #3=w540:i32, element #4=w539:i32)
        n231 = Index Array(array=w575, index=w562) -> (element=w576:T14)
        n232 = Index Array(array=w579, index=w562) -> (element=w578:T15)
        n233 = Unbundle By Name(w578) -> ("Wavelengths"=w566:dbl[])  [unwired: 1 out]
        n234 = Bundle By Name(cluster=w576, "Integration Time (ms)"=w542, "Optical Smoothing Level"=w541, "Number of Scans to Average"=w540, "Digitizer Clock Rate Setting"=w539, "Temp  Compensation"=w568) -> (w569:T14)
        n235 = call "StellarNet Set Parameters.vi"("Temp  Compensation"=w568, "Digitizer Clock Rate Setting"=w539, "error in (no error)"=w577, "Optical Smoothing Level"=w541, "Number of Scans to Average"=w540, "Integration Time (ms)"=w542) -> ("error out"=w567:errorcluster)  [unwired: 5 in]
        n236 = Replace Array Subset(array=w575, new element=w569, index=w562) -> ()  [unwired: 1 out]
        n237 = call "StellarNet Scan.vi"("error in (no error)"=w567, "Integration Time (msec)"=w542, "Spectral Channel"=w564) -> ("error out"=w588:errorcluster, "Critical Error"=w589:bool, "output param"=→"output param":i32)  [unwired: 5 in, 1 out]
        n238 = case shown="False" w589 {
          selector: w589 -> [_ w600]
          tunnel: w564 -> [w597 _]
          tunnel: [w596 w599] -> w573
          tunnel: [w594 w600] -> w586
          tunnel: w588 -> [w593 w598]
          tunnel: [w592 w598] -> w563
          tunnel: w542 -> [w591 _]
          frame False {
            n239 = call "StellarNet Scan.vi"("error in (no error)"=w593, "Integration Time (msec)"=w591, "Spectral Channel"=w597) -> ("error out"=w592:errorcluster, "buffer out"=w596:sgl[], "Critical Error"=w594:bool, "output param"=w595:i32)  [unwired: 5 in]
            n240 = local write "output param"(w595) -> ()
          }
          frame True {
            w599 = sgl[] []  # buffer out
            # "Critical Error"
          }
        }
        "Critical Error" <- w586
        n241 = Get Date/Time In Seconds() -> (seconds since 1Jan1904=w557:timestamp)
        n242 = Format Date/Time String(time format string (%c)="%Y-%m-%d %H_%M_%S", seconds (now)=w557) -> (date/time string=w552:string)  [unwired: 1 in]
        n243 = Split 1D Array(array=w573, index=2047) -> (first subarray=w565:sgl[])  [unwired: 1 out]
        n244 = Concatenate Strings(w552, ".txt") -> (w553:string)
        n245 = call <vilib>:"Simple Error Handler.vi"("error in (no error)"=w563) -> ()  [unwired: 4 in, 5 out]
        n246 = Build Array("wavelength (nm)", "intensity (a.u.)", w552) -> (w548:string[])
        n247 = Bundle("Wavelengths"=w566, w565) -> (→"Spectrum":cluster{"Wavelengths":dbl[], sgl[]})  [unwired: 1 in]
        n248 = Build Array(w566, w565) -> (w551:dbl[][])
        n249 = Build Path(base path="Save spectra file path", name or relative path=w553) -> (appended path=w555:path)
        n250 = Transpose 2D Array(2D array=w551) -> (transposed array=w550:dbl[][])
        n251 = call-poly <vilib>:"Write To Spreadsheet File.vi"("1D data"=w548, "file path (dialog if empty)"=w555) -> ("new file path (Not A Path if cancelled)"=w549:path)  [unwired: 6 in]
        n252 = call-poly <vilib>:"Write To Spreadsheet File.vi"("append to file? (new file:F)"=TRUE, "2D data"=w550, "file path (dialog if empty)"=w549) -> ()  [unwired: 5 in, 1 out]
      }
    }
    n253 = Multiply(x=u32 1000, y="Delay between data points (s)") -> (x*y=w321:dbl)
    n254 = Wait (ms)(milliseconds to wait=w321) -> ()  [unwired: 1 out]
    n255 = Equal To 0?(x=w314) -> (x = 0?=w305:bool)
    n256 = case "SRS QCM" shown="True" w404 {
      selector: w404 -> [w802 w807]
      tunnel: w406 -> [w805 w811]
      tunnel: w405 -> [w804 w812]
      tunnel: [w801 w818] -> w285
      tunnel: [w801 w817] -> w290
      tunnel: [w803 w816] -> w399
      tunnel: w350 -> [_ w815]
      tunnel: [w799 w814] -> w349
      tunnel: [w801 w813] -> w291
      tunnel: [T1 {"Numeric Control"=0.0, "Resistance out"=0.0} ("Cluster") w809] -> w326
      tunnel: [w799 w808] -> w325
      tunnel: w305 -> [_ w806]
      frame False {
        w799 = 0.0
        w801 = ""
        n257 = Bundle(w802, "VISA out"=w805, "error out"=w804) -> (w803:T16)  [unwired: 1 in]
      }
      frame True {
        # "SRS QCM"
        n258 = call "SRS_QCM_SubVI.vi"("VISA Refnum in"=w811, "first iteration?"=w806, "Frequency out 3"=w815, "Boolean 2"=w807, "Gate time"="Gate time", "error in (no error)"=w812) -> ("Frequency out 2"=w814:dbl, "Cluster"=w809:T1, "Frequency out"=w808:dbl, "Cluster 2"=w816:T17, "M"=w813:string, "MR"=w817:string, "F"=w818:string)  [unwired: 3 in]
      }
    }
    "Waveform Chart 2" <- w326
    "Hz" <- w325
    n259 = case "Setnag O2 Pump" shown="True" w398 {
      tunnel: [w822 w828] -> w410
      tunnel: w409 -> [w822 w829]
      tunnel: w321 -> [_ w825]
      tunnel: w403 -> [_ w827]
      tunnel: ["" w826] -> w402
      tunnel: [dbl[] [] w824] -> w324
      tunnel: [cluster{dbl} {0.0} w823] -> w323
      frame False {
      }
      frame True {
        # "SetNag O2 pump"
        n260 = call "setnag_o2_gauge_subVI.vi"("Numeric Control 3"=w829, "Com Port"=w827, "Numeric Control in"=w825) -> ("Cluster"=w823:cluster{"Numeric Control":dbl}, "Numeric Control out"=w828:dbl, "Array"=w824:dbl[], "String"=w826:string)  [unwired: 5 in]
      }
    }
    "appended array" <- w324
    "Waveform Chart" <- w323
    n261 = Bundle("M"=w291, "F"=w285, "MR"=w290) -> (w289:cluster{"M":string, "F":string, "MR":string})  [unwired: 1 in]
    n262 = Divide(x=w335, y=60.0) -> (x/y=w333:dbl)
    "Elapsed (min)" <- w333
    n263 = case "Keithley 2420" shown="True" w384 {
      selector: w384 -> [w788 w796]
      tunnel: w408 -> [w787 w791]
      tunnel: w407 -> [w786 w790]
      tunnel: [w785 w794] -> w400
      tunnel: ["" w793] -> w401
      frame False {
        n264 = Bundle(w788, "VISA resource name out"=w787, "error out"=w786) -> (w785:T10)  [unwired: 1 in]
      }
      frame True {
        # "Keithley 2420"
        n265 = call-poly "Read.vi"("VISA resource name"=w791, "error in (no error)"=w790) -> ("VISA resource name out"=w797:refnum<visa-resource-name>, "Resistance"=w792:sgl, "error out"=w795:errorcluster)  [unwired: 7 in, 4 out]
        n266 = Bundle("Resistance"=w792) -> (→"Keithley 2420 (Ohm)":cluster{"Resistance":sgl})  [unwired: 1 in]
        n267 = Number To Engineering String(4:w792) -> (0:w793:string)  [unwired: 3 in]
        n268 = Bundle(w796, "VISA resource name out"=w797, "error out"=w795) -> (w794:T10)  [unwired: 1 in]
      }
    }
    n269 = case "Keithley 6430" shown="False" w379 {
      selector: w379 -> [w764 w774]
      tunnel: w382 -> [w763 w771]
      tunnel: w381 -> [w762 w770]
      tunnel: ["" w773] -> w347
      tunnel: [w761 w772] -> w380
      frame False {
        n270 = Bundle(w764, "VISA resource name out"=w763, "error out"=w762) -> (w761:T10)  [unwired: 1 in]
      }
      frame True {
        # "Keithley 6430"
        n271 = call-poly "Read.vi"("error in (no error)"=w770, "VISA resource name"=w771) -> ("error out"=w769:errorcluster, "Measurement"=w767:dbl, "VISA resource name out"=w768:refnum<visa-resource-name>)  [unwired: 1 in, 6 out]
        n272 = Bundle("Measurement"=w767) -> (→"Keithley 6430 (Ohm)":cluster{"Measurement":dbl})  [unwired: 1 in]
        n273 = Number To Engineering String(4:w767) -> (0:w773:string)  [unwired: 3 in]
        n274 = Bundle(w774, "VISA resource name out"=w768, "error out"=w769) -> (w772:T10)  [unwired: 1 in]
      }
    }
    n275 = Select(t=w333, s=w336, f=w334) -> (s? t:f=w332:dbl)
    n276 = Greater Or Equal?(x=w333, y="Start saving after") -> (x >= y?=w346:bool)
    n277 = call "timing_and_saving_subVI.vi"("stop"="stop", "hrs"="hrs", "Data saving"="Data saving", "Auto stop after"="Auto stop after", "Numeric Control 3"=w333, "time to start saving?"=w346, "elapsed minutes"=w332, "Run Sequence"=w329, "arduinos ready?"=w322) -> ("STOP EVERYTHING"=w348:bool, "currently saving"=w272:bool, "save elapsed time"=w283:string)  [unwired: 4 in]
    "Currently saving data" <- w272
    n278 = Get Date/Time In Seconds() -> (seconds since 1Jan1904=w411:timestamp)
    n279 = Unbundle(w289) -> ("M"=w288:string, "F"=w287:string, "MR"=w286:string)
    n280 = Format Date/Time String(time format string (%c)="%Y-%m-%d %H:%M:%S%2u", seconds (now)=w411) -> (date/time string=w284:string)  [unwired: 1 in]
    n281 = Build Array(w284, w283, w347, w395, w401, w288, w287, w286, w402, w388, w372, w358, w371, w370) -> (w361:string[])
    n282 = Bundle("date/time string"=w284, "save elapsed time"=w283) -> (w282:T18)  [unwired: 1 in]
    n283 = Unbundle(w282) -> ("date/time string"=w281:string, "save elapsed time"=w280:string)
    n284 = Build Array(w281, w280, w279, w278, w277, w276, w275, w274) -> (w273:string[])
  }
  n285 = case shown="True" w28 {
    tunnel: w24 -> [_ w864]
    tunnel: w23 -> [_ w863]
    tunnel: w20 -> [_ w855]
    tunnel: w19 -> [_ w854]
    tunnel: w16 -> [_ w849]
    tunnel: w15 -> [_ w848]
    tunnel: w7 -> [_ w842]
    tunnel: w6 -> [_ w843]
    tunnel: w5 -> [_ w841]
    tunnel: w4 -> [_ w840]
    tunnel: w3 -> [_ w837]
    tunnel: w2 -> [_ w836]
    tunnel: w1 -> [_ w830]
    frame False {
    }
    frame True {
      w838 = T19 3 items=["no dialog", "OK message", "continue or stop message", "OK message + warnings", "continue/stop + warnings"] ("type of dialog (OK msg:1)")
      w845 = T19 3 items=["no dialog", "OK message", "continue or stop message", "OK message + warnings", "continue/stop + warnings"] ("type of dialog (OK msg:1)")
      w844 = T19 3 items=["no dialog", "OK message", "continue or stop message", "OK message + warnings", "continue/stop + warnings"] ("type of dialog (OK msg:1)")
      w850 = T19 3 items=["no dialog", "OK message", "continue or stop message", "OK message + warnings", "continue/stop + warnings"] ("type of dialog (OK msg:1)")
      w856 = T19 3 items=["no dialog", "OK message", "continue or stop message", "OK message + warnings", "continue/stop + warnings"] ("type of dialog (OK msg:1)")
      w858 = T19 3 items=["no dialog", "OK message", "continue or stop message", "OK message + warnings", "continue/stop + warnings"] ("type of dialog (OK msg:1)")
      n286 = VISA Close(VISA resource name=w849, error in (no error)=w848) -> (error out=w851:errorcluster)
      n287 = VISA Close(VISA resource name=w855, error in (no error)=w854) -> (error out=w857:errorcluster)
      n288 = VISA Close(VISA resource name=w863, error in (no error)=w864) -> (error out=w865:errorcluster)
      n289 = VISA Close(VISA resource name=w843, error in (no error)=w842) -> (error out=w847:errorcluster)
      n290 = call <vilib>:"Simple Error Handler.vi"("type of dialog (OK msg:1)"=w850, "error in (no error)"=w851) -> ()  [unwired: 3 in, 5 out]
      n291 = VISA Close(VISA resource name=w837, error in (no error)=w836) -> (error out=w839:errorcluster)
      n292 = call <vilib>:"Simple Error Handler.vi"("type of dialog (OK msg:1)"=w856, "error in (no error)"=w857) -> ()  [unwired: 3 in, 5 out]
      n293 = VISA Close(VISA resource name=w841, error in (no error)=w840) -> (error out=w846:errorcluster)
      n294 = call <vilib>:"Simple Error Handler.vi"("type of dialog (OK msg:1)"=w858, "error in (no error)"=w865) -> ()  [unwired: 3 in, 5 out]
      n295 = call <vilib>:"Simple Error Handler.vi"("type of dialog (OK msg:1)"=w844, "error in (no error)"=w847) -> ()  [unwired: 3 in, 5 out]
      n296 = call <vilib>:"Simple Error Handler.vi"("type of dialog (OK msg:1)"=w838, "error in (no error)"=w839) -> ()  [unwired: 3 in, 5 out]
      n297 = call <vilib>:"Simple Error Handler.vi"("type of dialog (OK msg:1)"=w845, "error in (no error)"=w846) -> ()  [unwired: 3 in, 5 out]
      n298 = Build Array("Date/Time" ("element"), "elapsed min" ("element"), "Filtered QCM 1" ("element"), "Filtered QCM 2" ("element"), "Filtered QCM 3" ("element"), "Filtered QCM4" ("element"), "Filtered QCM 5" ("element"), "Filtered QCM 6" ("element")) -> (w861:string[])
      n299 = call-poly <vilib>:"Write To Spreadsheet File.vi"("1D data"=w861) -> ("new file path (Not A Path if cancelled)"=w860:path)  [unwired: 7 in]
      n300 = call-poly <vilib>:"Write To Spreadsheet File.vi"("append to file? (new file:F)"=TRUE, "2D data"=w830, "file path (dialog if empty)"=w860) -> ()  [unwired: 5 in, 1 out]
    }
  }
  n301 = Unbundle(w120) -> ("Boolean"=w119:bool, "VISA out"=w118:refnum<visa-resource-name>, "error out"=w117:errorcluster)
  n302 = case shown="False" w119 {
    tunnel: w117 -> [w866 w869]
    tunnel: [w866 w868] -> w126
    tunnel: w118 -> [_ w867]
    frame False {
    }
    frame True {
      n303 = call "srsQcm200Close.vi"("error in"=w869, "Visa in"=w867) -> ("error out"=w868:errorcluster)  [unwired: 3 in]
    }
  }
  n304 = Unbundle(w124) -> (w123:bool, "VISA resource name out"=w122:refnum<visa-resource-name>, "error out"=w121:errorcluster)
  n305 = Unbundle(w115) -> ("Boolean"=w114:bool, "VISA resource name out"=w113:refnum<visa-resource-name>, "error out"=w112:errorcluster)
  n306 = case shown="True" w79 {
    tunnel: [w870 w888] -> w77
    tunnel: w80 -> [_ w887]
    tunnel: w81 -> [_ w886]
    tunnel: w83 -> [_ w882]
    tunnel: w82 -> [_ w881]
    tunnel: [w870 w880] -> w78
    tunnel: [w871 w877] -> w76
    tunnel: w75 -> [w871 w876]
    tunnel: w67 -> [_ w875]
    tunnel: [w870 w874] -> w70
    tunnel: w69 -> [_ w873]
    tunnel: w68 -> [_ w872]
    frame False {
      w870 = errorcluster {"status"=FALSE, "code"=0, "source"=""} ("error out")
    }
    frame True {
      n307 = disable-structure shown="Disabled" {
        disable-tunnel: [w892 _] -> w874
        disable-tunnel: w873 -> [w891 _]
        disable-tunnel: w872 -> [w890 _]
        frame Disabled {
          n308 = call <vilib>:"DAQmx Stop Task.vi"("task/channels in"=w891, "error in"=w890) -> ("task out"=w893:refnum<k21>, "error out"=w894:errorcluster)  [unwired: 12 in]
          n309 = call <vilib>:"DAQmx Clear Task.vi"("task in"=w893, "error in"=w894) -> ("error out"=w892:errorcluster)  [unwired: 13 in]
        }
        frame Enabled {
        }
      }
      n310 = call <vilib>:"DAQmx Stop Task.vi"("task/channels in"=w882, "error in"=w881) -> ("task out"=w884:refnum<k21>, "error out"=w883:errorcluster)  [unwired: 12 in]
      n311 = call <vilib>:"DAQmx Stop Task.vi"("task/channels in"=w887, "error in"=w886) -> ("task out"=w885:refnum<k21>, "error out"=w889:errorcluster)  [unwired: 12 in]
      n312 = VISA Clear(VISA resource name=w875, error in (no error)=w876) -> (VISA resource name out=w879:refnum<visa-resource-name>, error out=w878:errorcluster)
      n313 = call <vilib>:"DAQmx Clear Task.vi"("task in"=w884, "error in"=w883) -> ("error out"=w880:errorcluster)  [unwired: 13 in]
      n314 = call <vilib>:"DAQmx Clear Task.vi"("task in"=w885, "error in"=w889) -> ("error out"=w888:errorcluster)  [unwired: 13 in]
      n315 = VISA Close(VISA resource name=w879, error in (no error)=w878) -> (error out=w877:errorcluster)
    }
  }
  n316 = Unbundle(w87) -> (w92:bool, "VISA resource name out"=w91:refnum<visa-resource-name>, "error out"=w90:errorcluster)
  n317 = case shown="True" w123 {
    tunnel: w122 -> [_ w898]
    tunnel: w121 -> [w895 w897]
    tunnel: [w895 w896] -> w125
    frame False {
    }
    frame True {
      n318 = call "Enable Output.vi"("error in (no error)"=w897, "Enable Output (T: Enable)"=FALSE, "VISA resource name"=w898) -> ("error out"=w899:errorcluster, "VISA resource name out"=w901:refnum<visa-resource-name>)  [unwired: 7 in]
      n319 = call "Close.vi"("error in (no error)"=w899, "VISA resource name"=w901) -> ("error out"=w896:errorcluster)  [unwired: 9 in]
    }
  }
  n320 = case shown="True" w92 {
    tunnel: w91 -> [_ w904]
    tunnel: w90 -> [w902 w903]
    tunnel: [w902 w905] -> w86
    frame False {
    }
    frame True {
      w908 = FALSE  # Output (F:Off)
      n321 = call "Enable Output.vi"("error in (no error)"=w903, "Enable Output (F:Off)"=w908, "VISA resource name"=w904) -> ("error out"=w906:errorcluster, "VISA resource name out"=w907:refnum<visa-resource-name>)  [unwired: 7 out]
      n322 = call "Close.vi"("error in (no error)"=w906, "VISA resource name"=w907) -> ("error out"=w905:errorcluster)  [unwired: 9 out]
    }
  }
  n323 = case shown="True" w114 {
    tunnel: w113 -> [_ w912]
    tunnel: w112 -> [w909 w911]
    tunnel: [w909 w910] -> w111
    frame False {
    }
    frame True {
      n324 = VISA Close(VISA resource name=w912, error in (no error)=w911) -> (error out=w910:errorcluster)
    }
  }
  n325 = Merge Errors(w70, w78, w77, w76) -> (w54:errorcluster)
  n326 = Merge Errors(w53, w54) -> (w55:errorcluster)
  n327 = call <vilib>:"Simple Error Handler.vi"("error in (no error)"=w55) -> ()  [unwired: 4 in, 5 out]
  n328 = Merge Errors(w86, w111, w125, w126) -> (w132:errorcluster)
  n329 = call <vilib>:"Simple Error Handler.vi"("error in (no error)"=w132) -> ()  [unwired: 4 in, 5 out]
  n330 = Build Array("date/time", "min elapsed", "Keithley 6430 R (Ohm)", "J-KEM temp (C)", "Keithley 2420 R (Ohm)" ("element"), "QCM mass (ug)", "QCM f (Hz)", "QCM R (Ohm)", "O2 PP (Torr)" ("element"), "O2 conc (PPM)" ("element"), "pressure (Torr)" ("element"), "RH (%)" ("element"), "gas flow (sccm)" ("element"), "vapor flow (sccm)" ("element"), "first filter" ("element"), "second filter" ("element"), "raw qcm data" ("element"), "Experiment Notes") -> (w103:string[])
  n331 = call-poly <vilib>:"Write To Spreadsheet File.vi"("1D data"=w103, "file path (dialog if empty)"=w96) -> ("new file path (Not A Path if cancelled)"=w104:path)  [unwired: 6 in]
  n332 = call-poly <vilib>:"Write To Spreadsheet File.vi"("append to file? (new file:F)"=TRUE, "2D data"=w30, "file path (dialog if empty)"=w104) -> ()  [unwired: 5 in, 1 out]
